vi "Steuerprogramm03-15.vi"() -> ()   [LabVIEW 2010]
uses:
  <vilib>/rvi/interface/nirviReadWriteControl/nirviReadWriteControl.xnode
  <vilib>/rvi/errors/niLvFpgaWhatHappensToTopLevelVI.ctl
  <vilib>/rvi/interface/common/niFpgaNodeNameForErrorReporting.ctl
  <vilib>/rvi/errors/niLvFpgaAdjustHostInterfaceError.vi
  gvbooleschRT.vi
  <vilib>/functionblocks/FB Core/FB Core.xnode
  <vilib>/functionblocks/Counter/Elapsed Timer/Elapsed Timer.vi
  <vilib>/functionblocks/NI_FunctionBlock Libraries.lvlib
  <vilib>/rvi/interface/nirviCloseFPGA/nirviCloseFPGA.xnode
  <vilib>/addons/control/pid/NI_PID_pid.lvlib
  C:/Users/HAGAR-IV/Desktop/Zeugs/Johnny/pertrasgc fpga/FPGA-Programm-10-14.vi
  C:/Users/HAGAR-IV/Desktop/Zeugs/markus/version feb 2012/FPGA Bitfiles/pertrasgcfpga2_FPGATarget_FPGA-Programm-10_16368CB6.lvbitx
  GVMWHorst.vi
  GVMethodenwechsel.vi
  GVHorstSP.vi
  GVZwangs.vi
  GVHK1Hz.vi
  GVHeizenLH.vi
  GVAIs.vi
  <vilib>/addons/control/pid/pid.llb/PID (DBL Array).vi
  GVTrapsMachs.vi
  GVaktuelleTDMS.vi
  GVECDs.vi
  GVZeitenZyklen.vi
  GVProbenvol.vi
  GVVentilposition.vi
  NiFpgaLv.dll
  <vilib>/Utility/error.llb/Error Cluster From Error Code.vi
  <vilib>/Instr/_visa.llb/VISA Configure Serial Port (Instr).vi
  <vilib>/rvi/interface/nirviMethod/nirviMethod.xnode
  GVChroms.vi
  <vilib>/FPGAPlugInAG/cRIO-9114/niLvFpga_Close_cRIO-9114.vi
panel:
  out "AIs3":dbl[](array[numeric])
  out "AIs2":dbl[](array[numeric])
  in  "Tabellarische Darstellung":bool
  out "AIs3":string[](array[string])
  out "AIs2":string[](array[string])
  out "AIs1":string[](array[string])
  out "AIs1":dbl[](array[numeric])
  in  "ServosWarmHigh (us)KaltHigh(us)":T1
  in  "An/Aus":bool
  in  "dargestellte Größe 3":i32(ring)=1 items=["U_WiderstandTrap1 [V]", "TemperaturTrap1 [°C]", "U_WiderstandTrap2 [V]", "TemperaturTrap2 [°C]", "TemperaturMach1 [°C]", "TemperaturMach2 [°C]", "PrC0", "PrC1-Säule2", "PrC1-Säule1", "MFC1-Sample", "MFC1-Methan", "PrC1-BackFlush1", "PrC1-BackFlush2", "MFC2A", "MFC2B", "MFC2C", "PrC2A", "PrC2C", "MFC2D", "MFC2E", "PrC2B"]
  in  "TafelWischen!":bool
  out "schnelleAnzeige":cluster{dbl[], dbl[]}(graph)
  in  "senden":bool
  in  "Schreibpuffer":string
  out "vomLicor":string
  in  "Licor":bool
  in  "SerielleKomm.":bool=TRUE
  in  "ECDSpeichern":bool=TRUE
  in  "HKSpeichern":bool
  in  "Methode speichern":bool
  in  "DetYMax":dbl=100.0
  in  "DetYMin":dbl
  in  "HK2YMax":dbl=100.0
  in  "HK2YMin":dbl
  in  "HK1YMax":dbl=100.0
  in  "HK1YMin":dbl
  out "ZyklusNummernGesamt":i32[](array[numeric])
  in  "Detektor":i32(ring) items=["ECD1", "ECD2"]
  out "Detektor":cluster{dbl[], dbl[]}[](graph)
  out "Zykluslängen [s]":dbl[](array[numeric])
  in  "veränderte Methode benutzen":bool
  in  "Methode verändern":bool
  in  "dargestellte Größe 2":i32(ring)=1 items=["T1-Trap1", "T1-Trap2", "T1-StirlingKühlkopf", "T1-PreCol1", "T1-PreCol2", "T1-MainCol1a", "T1-MainCol1b", "T1-MainCol2a", "T1-MainCol2b", "T1-Bronkhorst1a", "T1-Bronkhorst1b", "T1-Bronkhorst2a", "T1-Bronkhorst2b", "T1-2Pos1B", "T1-Spare9", "T1-2Pos1A", "T1-Spare10", "T1-TurboPump", "T1-StirlingPlatine", "T1-Spare5", "T1-Spare6", "T1-Spare7", "T1-Spare8", "F1-MFM1", "F1-MFM2", "P1-MethaneHP", "P1-MethaneLP", "P1-Vacuum", "TurboSpeed", "I1-MS-AC", "I1-Trap1", "I1-Trap2", "T2-ECD1a", "T2-ECD1b", "T2-ECD2a", "T2-ECD2b", "T2-Col1a", "T2-Col1b", "T2-Col2a", "T2-Col2b", "T2-Spare1", "T2-Spare2", "T2-Oven_a", "T2-Oven_b", "T2-Spare3", "T2-Spare4", "T2-Spare5", "F2-MFM0", "F2-MFM2A", "F2-MFM2B", "P2-N2O_HP", "P2-N2O_LP", "P2-CO2_HP", "P2-CO2_LP", "AI-Spare1", "AI-Spare2", "AI-Spare3", "AI-Spare4", "AI-Spare5", "AI-Spare6", "AI-Spare7", "AI-Spare8", "AI-Spare9", "AI-Spare10", "T0-DC/DC5", "I0-24V_M0", "I0-48V_M1", "I0-24V_M1", "I0-28V_M2", "T0-Drier", "T0-Spare2", "T0-Spare4", "T0-DC/DC7", "I0-20V_Laptop", "I0-28V_M1", "I0-24V_M2", "I0-12V_Licor", "T0-Spare1", "T0-Spare3", "T0-Spare5", "F0-MFM1", "TL-Licor_a", "P0-NitrogenHP", "P0-HeliumHP", "P0-Standard1HP", "P0-Standard2HP", "P0-Standard3HP", "AI-Spare11", "F0-MFM2", "TL-Licor_b", "P0-NitrogenLP", "P0-HeliumLP", "P0-Standard1LP", "P0-Standard2LP", "P0-Standard3LP", "AI-Spare12", "U_WiderstandTrap1 [V]", "TemperaturTrap1 [°C]", "U_WiderstandTrap2 [V]", "TemperaturTrap2 [°C]", "TemperaturMach1 [°C]", "TemperaturMach2 [°C]", "PrC0", "PrC1-Säule2", "PrC1-Säule1", "MFC1-Sample", "MFC1-Methan", "PrC1-BackFlush1", "PrC1-BackFlush2", "MFC2A", "MFC2B", "MFC2C", "PrC2A", "PrC2C", "MFC2D", "MFC2E", "PrC2B"]
  in  "Zeitachse2":i32(ring)=1 items=["Zykluszeit [s] Mod0", "Zykluszeit [s] Mod1", "Zykluszeit [s] Mod2A", "Zykluszeit [s] Mod2B"]
  out "Housekeeping2":cluster{dbl[], dbl[]}(graph)
  out "ZyklusNummern":i32[](array[numeric])
  in  "dargestellte Größe 1":i32(ring)=1 items=["T1-Trap1", "T1-Trap2", "T1-StirlingKühlkopf", "T1-PreCol1", "T1-PreCol2", "T1-MainCol1a", "T1-MainCol1b", "T1-MainCol2a", "T1-MainCol2b", "T1-Bronkhorst1a", "T1-Bronkhorst1b", "T1-Bronkhorst2a", "T1-Bronkhorst2b", "T1-2Pos1B", "T1-Spare9", "T1-2Pos1A", "T1-Spare10", "T1-TurboPump", "T1-StirlingPlatine", "T1-Spare5", "T1-Spare6", "T1-Spare7", "T1-Spare8", "F1-MFM1", "F1-MFM2", "P1-MethaneHP", "P1-MethaneLP", "P1-Vacuum", "TurboSpeed", "I1-MS-AC", "I1-Trap1", "I1-Trap2", "T2-ECD1a", "T2-ECD1b", "T2-ECD2a", "T2-ECD2b", "T2-Col1a", "T2-Col1b", "T2-Col2a", "T2-Col2b", "T2-Spare1", "T2-Spare2", "T2-Oven_a", "T2-Oven_b", "T2-Spare3", "T2-Spare4", "T2-Spare5", "F2-MFM0", "F2-MFM2A", "F2-MFM2B", "P2-N2O_HP", "P2-N2O_LP", "P2-CO2_HP", "P2-CO2_LP", "AI-Spare1", "AI-Spare2", "AI-Spare3", "AI-Spare4", "AI-Spare5", "AI-Spare6", "AI-Spare7", "AI-Spare8", "AI-Spare9", "AI-Spare10", "T0-DC/DC5", "I0-24V_M0", "I0-48V_M1", "I0-24V_M1", "I0-28V_M2", "T0-Drier", "T0-Spare2", "T0-Spare4", "T0-DC/DC7", "I0-20V_Laptop", "I0-28V_M1", "I0-24V_M2", "I0-12V_Licor", "T0-Spare1", "T0-Spare3", "T0-Spare5", "F0-MFM1", "TL-Licor_a", "P0-NitrogenHP", "P0-HeliumHP", "P0-Standard1HP", "P0-Standard2HP", "P0-Standard3HP", "AI-Spare11", "F0-MFM2", "TL-Licor_b", "P0-NitrogenLP", "P0-HeliumLP", "P0-Standard1LP", "P0-Standard2LP", "P0-Standard3LP", "AI-Spare12", "U_WiderstandTrap1 [V]", "TemperaturTrap1 [°C]", "U_WiderstandTrap2 [V]", "TemperaturTrap2 [°C]", "TemperaturMach1 [°C]", "TemperaturMach2 [°C]", "PrC0", "PrC1-Säule2", "PrC1-Säule1", "MFC1-Sample", "MFC1-Methan", "PrC1-BackFlush1", "PrC1-BackFlush2", "MFC2A", "MFC2B", "MFC2C", "PrC2A", "PrC2C", "MFC2D", "MFC2E", "PrC2B"]
  in  "Zeitachse1":i32(ring)=1 items=["Zykluszeit [s] Mod0", "Zykluszeit [s] Mod1", "Zykluszeit [s] Mod2A", "Zykluszeit [s] Mod2B"]
  out "Housekeeping1":cluster{dbl[], dbl[]}(graph)
  out "Big Ben, Methodenzeit, Zykluszeit0, Zykluszeit1, Zykluszeit2A, Zykluszeit2B":i32[](array[numeric])
  in  "global stop RT":bool
  in  "Methode":i32(ring) items=["Leer"]
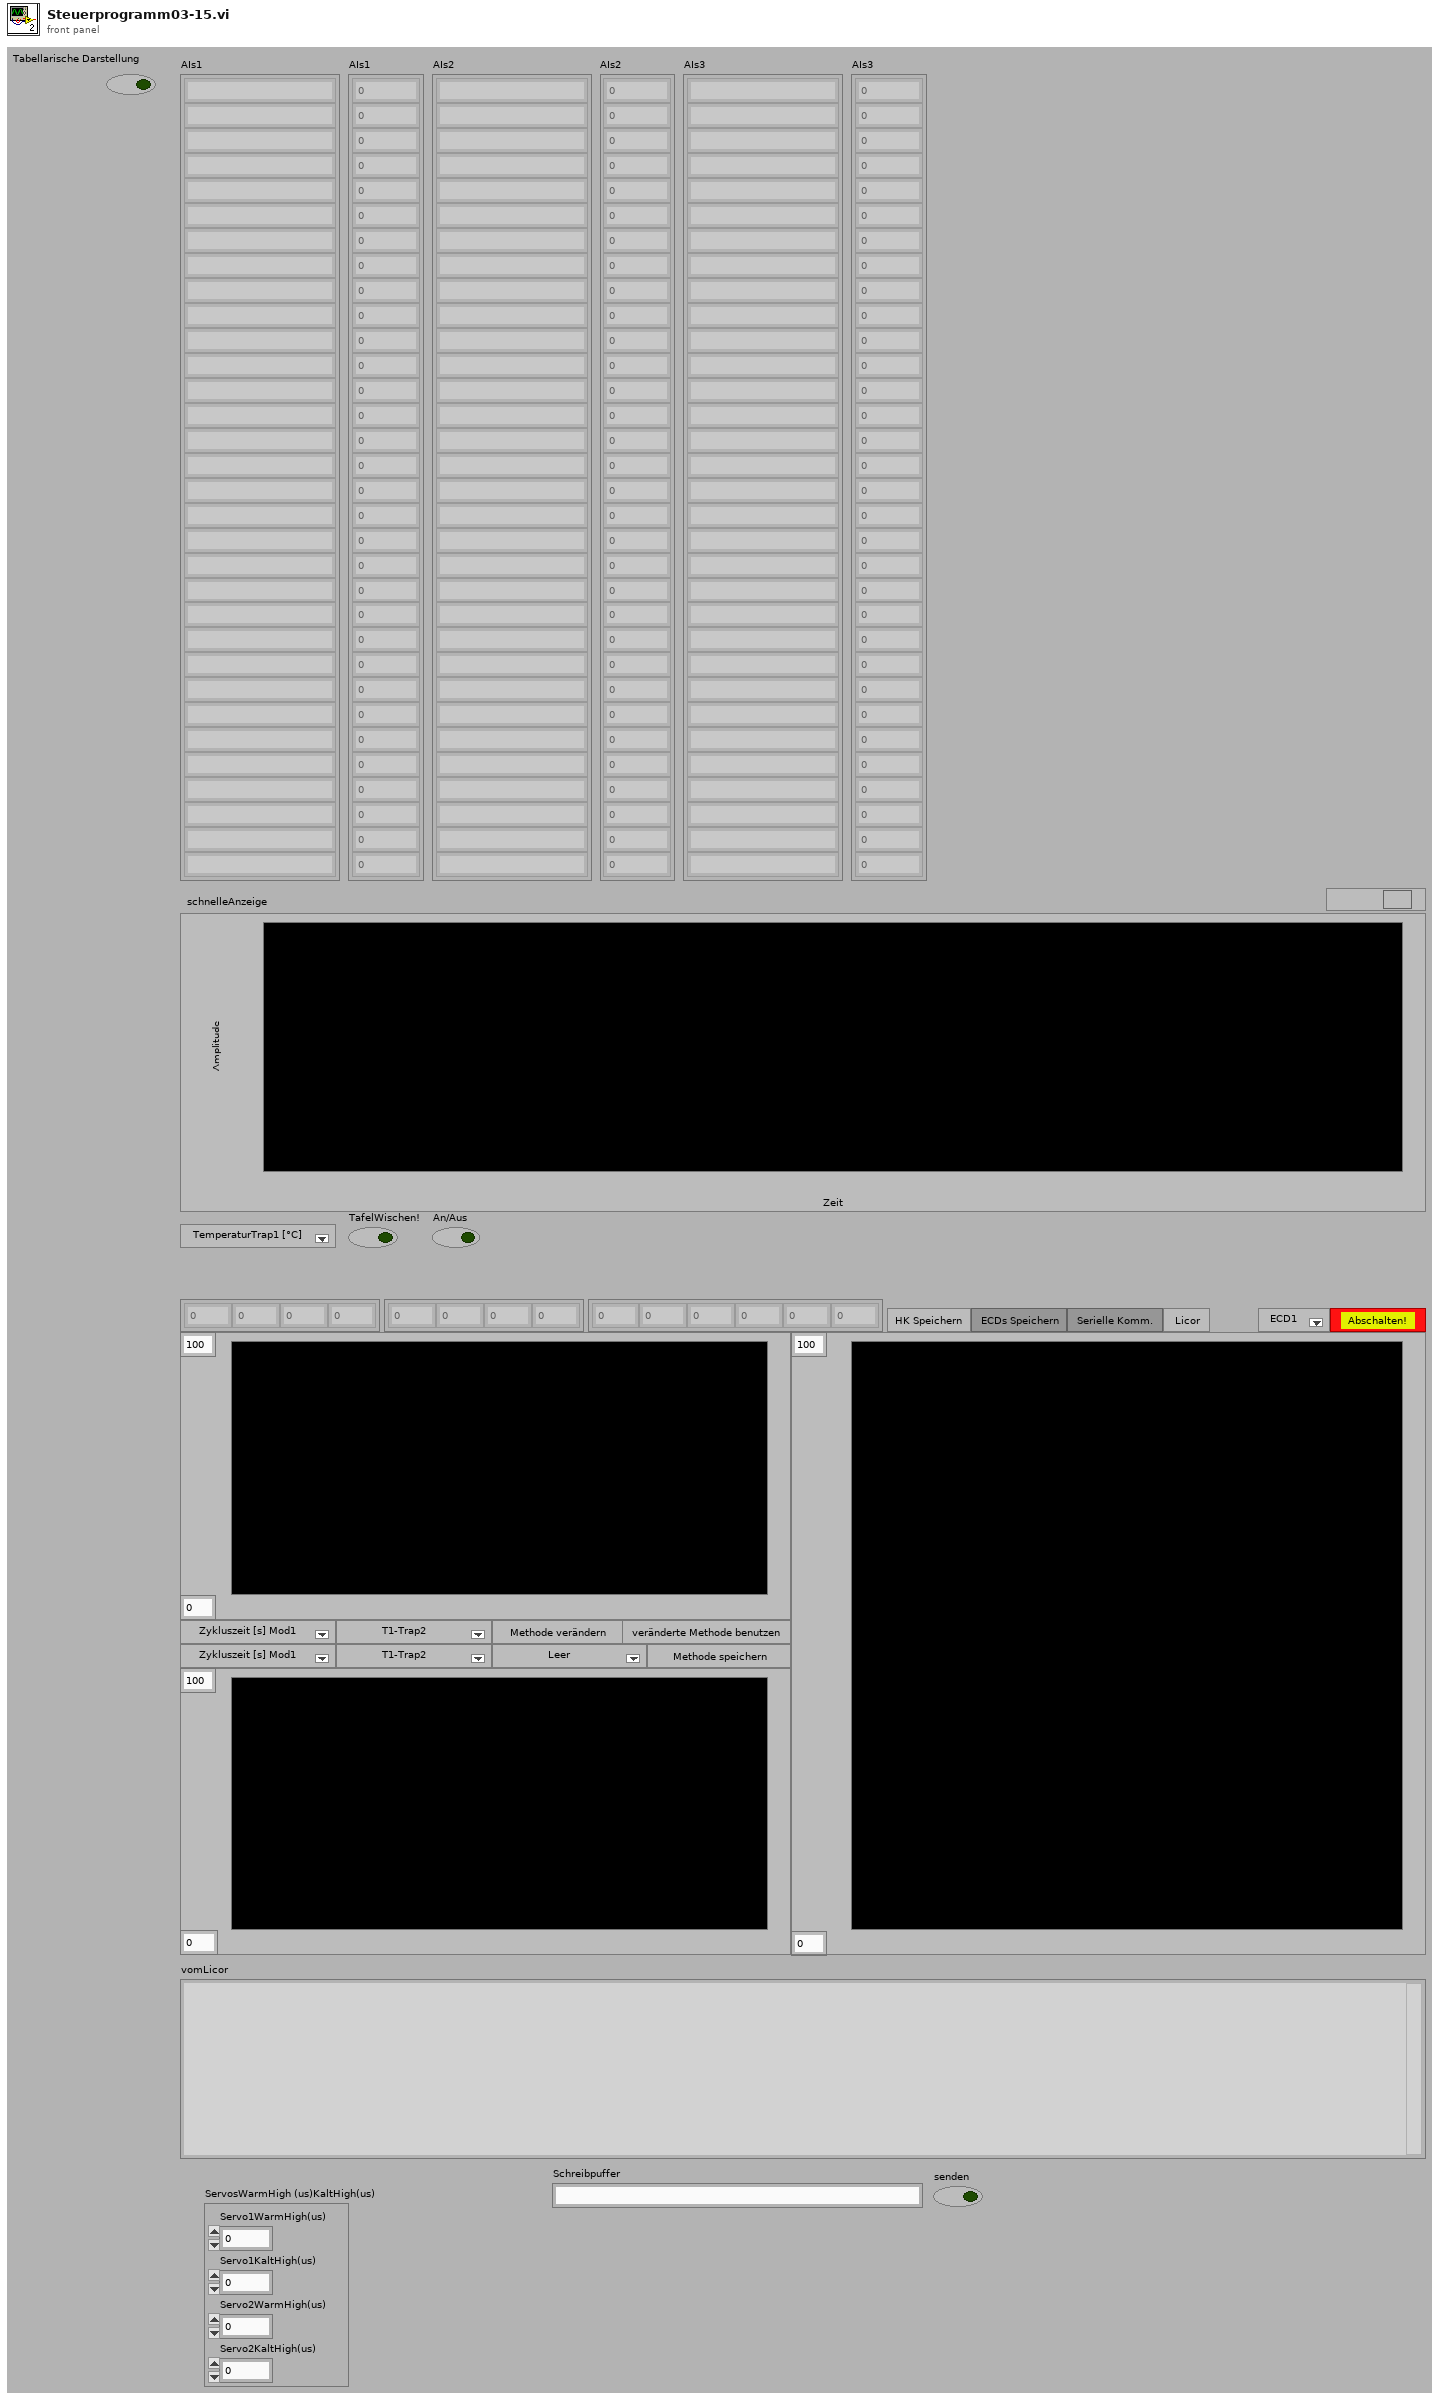
[diagram p1: front panel]
types:
  T1 = cluster{"Servo1WarmHigh(us)":u32, "Servo1KaltHigh(us)":u32, "Servo2WarmHigh(us)":u32, "Servo2KaltHigh(us)":u32}
  T2 = cluster{"Zykluslängen [s]":dbl[], "ZeitpktDIOsMod0":dbl[], "ZeitpktDIOsMod1":dbl[], "ZeitpktDIOsMod2A":dbl[], "ZeitpktDIOsMod2B":dbl[], "DIOsSPMod0":bool[][], "DIOsSPMod1":bool[][], "DIOsSPMod2A":bool[][], "DIOsSPMod2B":bool[][], "Mod0HorstZeitpkt":dbl[], "Mod1HorstZeitpkt":dbl[], "Mod2AHorstZeitpkt":dbl[], "Mod2BHorstZeitpkt":dbl[], "HorstSPMod0":dbl[][], "HorstSPMod1":dbl[][], "HorstSPMod2A":dbl[][], "HorstSPMod2B":dbl[][], "LangsameHeizungenSP":dbl[], "LHHeizen?":bool[], "ZPktFPGABoolesch":dbl[], "FPGABoolesch":bool[][], "ZeitpktFPGAPID":dbl[], "FPGAPID":cluster{"proportional gain (Kc)":fxp<+/-,16,8>, "integral gain (Kc*Ts/Ti)":fxp<+/-,16,8>, "derivative gain (Kc*Td/Ts)":fxp<+/-,16,8>}[][], "ZeitpktFPGAFixp":dbl[], "FPGAFixp":fxp<+/-,16,4>[][], "ZeitpktMach1":dbl[], "TempMach1":dbl[], "ZeitpktMach2":dbl[], "TempMach2":dbl[], "PIDs für \"träge\" Heizungen":cluster{"proportional gain (Kc)":dbl, "integral time (Ti, min)":dbl, "derivative time (Td, min)":dbl}[], "Zwangsbedingungen":dbl[][], "Dateien fürs MS schicken?":bool, "ZeitpunkteMPV":dbl[], "SPMPV":i32[], "ZeitpktMSa":dbl, "ZeitpktMSb":dbl, "Int.Start1":dbl, "Int.Stop1":dbl, "Int.Start2":dbl, "Int.Stop2":dbl, "Methodenname":string}[]
  T3 = cluster{"DIOsMod0Nr":i32[], "DIOsMod1Nr":i32[], "DIOsMod2ANr":i32[], "DIOsMod2BNr":i32[], "AIsLH":i32[], "Anzahl Horst/Modul":i32[], "Regler für den Probenfluß":i32, "StringSPvorgebenMod0":string[], "StringSPvorgebenMod1":string[], "StringSPvorgebenMod2A":string[], "StringSPvorgebenMod2B":string[], "StringMWAntwort0":string[], "StringMWAntwort1":string[], "StringMWAntwort2A":string[], "StringMWAntwort2B":string[], "UmrechnungHorst0":dbl[], "UmrechnungHorst1":dbl[], "UmrechnungHorst2A":dbl[], "UmrechnungHorst2B":dbl[], "StringMWabfragenMod0":string[], "StringMWabfragenMod1":string[], "StringMWabfragenMod2A":string[], "StringMWabfragenMod2B":string[], "Modul1/AI koeff":dbl[][], "Modul2/AI koeff":dbl[][], "Modul3/AI koeff":dbl[][], "Traps/MachsKoeff":dbl[][], "Modul1/AIsNamen":string[], "Modul2/AIsNamen":string[], "Modul3/AIsNamen":string[], "DIOsMod0Name":string[], "DIOsMod1Name":string[], "DIOsMod2AName":string[], "DIOsMod2BName":string[], "HorstMod0Name":string[], "HorstMod1Name":string[], "HorstMod2AName":string[], "HorstMod2BName":string[], "Startmethode":i32, "Dateiordner Housekeeping":path, "Dateiname Housekeeping":string, "DateiordnerECD1":path, "DateinameECD1":string, "DateiordnerECD2":path, "DateinameECD2":string, "NamenLangsameHeizungen":string[], "ModuleLH":i32[]}
  T4 = enum16{"open", "replace", "create", "open or create", "replace or create", "replace or create with confirmation"}
  T5 = cluster{"DIOsMod0Nr":i32[], "DIOsMod1Nr":i32[], "DIOsMod2ANr":i32[], "DIOsMod2BNr":i32[], "AIs für \"träge\" Heizungen":i32[], i32[], "AnschlüsseHorstMod0":enum8{"0", "1", "2", "3", "4", "5", "6", "7", "8"}[], "AnschlüsseHorstMod1":enum8{"0", "1", "2", "3", "4", "5", "6", "7", "8"}[], "AnschlüsseHorstMod2A":enum8{"0", "1", "2", "3", "4", "5", "6", "7", "8"}[], "AnschlüsseHorstMod2B":enum8{"0", "1", "2", "3", "4", "5", "6", "7", "8"}[], "StringSPvorgebenMod0":string[], "StringSPvorgebenMod1":string[], "StringSPvorgebenMod2A":string[], "StringSPvorgebenMod2B":string[], "StringMWAntwort0":string[], "StringMWAntwort1":string[], "StringMWAntwort2A":string[], "StringMWAntwort2B":string[], "UmrechnungHorst0":dbl[], "UmrechnungHorst1":dbl[], "UmrechnungHorst2A":dbl[], "UmrechnungHorst2B":dbl[], "StringMWabfragenMod0":string[], "StringMWabfragenMod1":string[], "StringMWabfragenMod2A":string[], "StringMWabfragenMod2B":string[], "Modul1/AI koeff":dbl[][], "Modul2/AI koeff":dbl[][], "Modul3/AI koeff":dbl[][], "Traps/MachKoeff":dbl[][], "AIsNamen":string[], "DIOsMod0Name":string[], "DIOsMod1Name":string[], "DIOsMod2AName":string[], "DIOsMod2BName":string[], "HorstMod0Name":string[], "HorstMod1Name":string[], "HorstMod2AName":string[], "HorstMod2BName":string[], "Startmethode":i32, "Dateiordner Housekeeping":path, "Dateiname Housekeeping":string, "DateiordnerECD1":path, "DateinameECD1":string, "DateiordnerECD2":path, "DateinameECD2":string}
  T6 = cluster{"Zykluslängen [s]":dbl[], "ZeitpktDIOsMod0":dbl[], "ZeitpktDIOsMod1":dbl[], "ZeitpktDIOsMod2A":dbl[], "ZeitpktDIOsMod2B":dbl[], "DIOsSPMod0":bool[][], "DIOsSPMod1":bool[][], "DIOsSPMod2A":bool[][], "DIOsSPMod2B":bool[][], "Mod0HorstZeitpkt":dbl[], "Mod1HorstZeitpkt":dbl[], "Mod2AHorstZeitpkt":dbl[], "Mod2BHorstZeitpkt":dbl[], "HorstSPMod0":dbl[][], "HorstSPMod1":dbl[][], "HorstSPMod2A":dbl[][], "HorstSPMod2B":dbl[][], "LangsameHeizungenSP":dbl[], "LHHeizen?":bool[], "ZPktFPGABoolesch":dbl[], "FPGABoolesch":bool[][], "ZeitpktFPGAPID":dbl[], "FPGAPID":cluster{"proportional gain (Kc)":fxp<+/-,16,8>, "integral gain (Kc*Ts/Ti)":fxp<+/-,16,8>, "derivative gain (Kc*Td/Ts)":fxp<+/-,16,8>}[][], "ZeitpktFPGAFixp":dbl[], "FPGAFixp":fxp<+/-,16,4>[][], "ZeitpktMach1":dbl[], "TempMach1":dbl[], "ZeitpktMach2":dbl[], "TempMach2":dbl[], "PIDs für \"träge\" Heizungen":cluster{"proportional gain (Kc)":dbl, "integral time (Ti, min)":dbl, "derivative time (Td, min)":dbl}[], "Zwangsbedingungen":dbl[][], "Text0 MS-Datei":string, "Info":string, "wie wird gespeichert?":u16, "Speicherlänge":string, "Dateien fürs MS schicken?":bool, "Pfad MS-Datei CRIO":path}[]
  T7 = cluster{"DIOsMod0Nr":i32[], "DIOsMod1Nr":i32[], "DIOsMod2ANr":i32[], "DIOsMod2BNr":i32[], "AIs für \"träge\" Heizungen":i32[], i32[], "AnschlüsseHorstMod0":enum8{"0", "1", "2", "3", "4", "5", "6", "7", "8"}[], "AnschlüsseHorstMod1":enum8{"0", "1", "2", "3", "4", "5", "6", "7", "8"}[], "AnschlüsseHorstMod2A":enum8{"0", "1", "2", "3", "4", "5", "6", "7", "8"}[], "AnschlüsseHorstMod2B":enum8{"0", "1", "2", "3", "4", "5", "6", "7", "8"}[], "StringSPvorgebenMod0":string[], "StringSPvorgebenMod1":string[], "StringSPvorgebenMod2A":string[], "StringSPvorgebenMod2B":string[], "StringMWAntwort0":string[], "StringMWAntwort1":string[], "StringMWAntwort2A":string[], "StringMWAntwort2B":string[], "UmrechnungHorst0":dbl[], "UmrechnungHorst1":dbl[], "UmrechnungHorst2A":dbl[], "UmrechnungHorst2B":dbl[], "StringMWabfragenMod0":string[], "StringMWabfragenMod1":string[], "StringMWabfragenMod2A":string[], "StringMWabfragenMod2B":string[], "Modul1/AI koeff":dbl[][], "Modul2/AI koeff":dbl[][], "Modul3/AI koeff":dbl[][], "Traps/MachKoeff":dbl[][], "AIsNamen":string[], "DIOsMod0Name":string[], "DIOsMod1Name":string[], "DIOsMod2AName":string[], "DIOsMod2BName":string[], "HorstMod0Name":string[], "HorstMod1Name":string[], "HorstMod2AName":string[], "HorstMod2BName":string[], "Startmethode":i32, "Dateiordner Housekeeping":path, "Dateiname Housekeeping":string}
  T8 = typedef "niFpgaNodeNameForErrorReporting.ctl" = enum16{"Open FPGA VI Reference", "Read/Write Control", "Invoke Method: Abort", "Invoke Method: Acknowledge IRQ", "Invoke Method: Download", "Invoke Method: FIFO.Configure", "Invoke Method: FIFO.Read", "Invoke Method: FIFO.Start", "Invoke Method: FIFO.Stop", "Invoke Method: FIFO.Write", "Invoke Method: Reset", "Invoke Method: Run", "Invoke Method: Wait on IRQ", "Close FPGA VI Reference"}
  T9 = typedef "niLvFpgaWhatHappensToTopLevelVI.ctl" = enum16{"top level VI scripted behind XNode", "top level VI inlined behind XNode"}
  T10 = cluster{"Zyklus1":i32, "Zeitachse1":i32, "dargestellte Größe 1":i32, "Zyklus2":i32, "Zeitachse2":i32, "dargestellte Größe 2":i32}
  T11 = cluster{"DIOsMod0Name":string[], "DIOsMod1Name":string[], "DIOsMod2AName":string[], "DIOsMod2BName":string[], "HorstMod0Name":string[], "HorstMod1Name":string[], "HorstMod2AName":string[], "HorstMod2BName":string[], "NamenLangsameHeizungen":string[]}
  T12 = cluster{"Dateiordner Housekeeping":path, "DateiordnerECD1":path, "DateiordnerECD2":path, "Dateiname Housekeeping":string, "DateinameECD1":string, "DateinameECD2":string, "tdms0":refnum<k34>, "tdms1":refnum<k34>, "tdms0":refnum<k34>, "tdms1":refnum<k34>, "tdms0":refnum<k34>, "tdms1":refnum<k34>}
  T13 = cluster{"Zykluslängen [s]":dbl[], "ZeitpktDIOsMod0":dbl[], "ZeitpktDIOsMod1":dbl[], "ZeitpktDIOsMod2A":dbl[], "ZeitpktDIOsMod2B":dbl[], "DIOsSPMod0":bool[][], "DIOsSPMod1":bool[][], "DIOsSPMod2A":bool[][], "DIOsSPMod2B":bool[][], "Mod0HorstZeitpkt":dbl[], "Mod1HorstZeitpkt":dbl[], "Mod2AHorstZeitpkt":dbl[], "Mod2BHorstZeitpkt":dbl[], "HorstSPMod0":dbl[][], "HorstSPMod1":dbl[][], "HorstSPMod2A":dbl[][], "HorstSPMod2B":dbl[][], "LangsameHeizungenSP":dbl[], "LHHeizen?":bool[], "ZPktFPGABoolesch":dbl[], "FPGABoolesch":bool[][], "ZeitpktFPGAPID":dbl[], "FPGAPID":cluster{"proportional gain (Kc)":fxp<+/-,16,8>, "integral gain (Kc*Ts/Ti)":fxp<+/-,16,8>, "derivative gain (Kc*Td/Ts)":fxp<+/-,16,8>}[][], "ZeitpktFPGAFixp":dbl[], "FPGAFixp":fxp<+/-,16,4>[][], "ZeitpktMach1":dbl[], "TempMach1":dbl[], "ZeitpktMach2":dbl[], "TempMach2":dbl[], "PIDs für \"träge\" Heizungen":cluster{"proportional gain (Kc)":dbl, "integral time (Ti, min)":dbl, "derivative time (Td, min)":dbl}[], "Zwangsbedingungen":dbl[][], "Dateien fürs MS schicken?":bool, "ZeitpunkteMPV":dbl[], "SPMPV":i32[], "ZeitpktMSa":dbl, "ZeitpktMSb":dbl, "Int.Start1":dbl, "Int.Stop1":dbl, "Int.Start2":dbl, "Int.Stop2":dbl, "Methodenname":string}
  T14 = cluster{"proportional gain (Kc)":fxp<+/-,16,8>, "integral gain (Kc*Ts/Ti)":fxp<+/-,16,8>, "derivative gain (Kc*Td/Ts)":fxp<+/-,16,8>}[][]
  T15 = cluster{"proportional gain (Kc)":dbl, "integral time (Ti, min)":dbl, "derivative time (Td, min)":dbl}[]
  T16 = cluster{"Heizen?LH[0]":bool, "Heizen?LH[1]":bool, "Heizen?LH[2]":bool, "Heizen?LH[3]":bool, "Heizen?LH[4]":bool, "Heizen?LH[5]":bool, "Heizen?LH[6]":bool, "Heizen?LH[7]":bool, "Heizen?LH[8]":bool, "Heizen?LH[9]":bool, "Heizen?LH[10]":bool, "Heizen?LH[11]":bool, "Heizen?LH[12]":bool, "Heizen?LH[13]":bool}
  T17 = cluster{"[0]":u32, "[1]":u32, "[2]":u32, "[3]":u32, "[4]":u32, "[5]":u32, "[6]":u32, "[7]":u32, "[8]":u32, "[9]":u32, "[10]":u32, "[11]":u32, "[12]":u32, "[13]":u32}
  T18 = cluster{cluster{"ZeitpktDIOsMod2B":dbl[]}[], cluster{"DIOsSPMod2B":bool[][]}[], cluster{"Mod2BHorstZeitpkt":dbl[]}[], cluster{"HorstSPMod2B":dbl[][]}[], "LHHeizen?":bool[], "ZPktFPGABoolesch":dbl[], "FPGABoolesch":bool[][], "ZeitpktFPGAPID":dbl[], "FPGAPID":cluster{"proportional gain (Kc)":fxp<+/-,16,8>, "integral gain (Kc*Ts/Ti)":fxp<+/-,16,8>, "derivative gain (Kc*Td/Ts)":fxp<+/-,16,8>}[][], "ZeitpktFPGAFixp":dbl[], "FPGAFixp":fxp<+/-,16,4>[][], "ZeitpktMach1":dbl[], "TempMach1":dbl[], "ZeitpktMach2":dbl[], "TempMach2":dbl[], "ZeitpunkteMPV":dbl[], "SPMPV":i32[]}
  T19 = cluster{"ZyklusNummern":i32[], "ZeilennummernDIOs":i32[], "ZwangsDIO?":cluster{bool[]}[], "ZeilennummernHorst":i32[], "ZwangsHorst?":cluster{bool[]}[], "ZeileFPGABoolesch":i32, "ZwangsFPGABoolesch?":bool[], "ZeileFPGAPID":i32, "ZeileFPGAFixp":i32, "ZeileMach1":i32, "ZeileMach2":i32, "ZeilennummerMPV":i32}
  T20 = cluster{"Zyklusnummern 0, 1, 2A, 2B":i32[], i32[], "ZwangsDIO?":cluster{bool[]}[], i32[], "ZwangsHorst?":cluster{bool[]}[], i32, "ZwangsFPGABoolesch?":bool[], i32, i32, i32, i32, "ZeilennummerMPV":i32}
  T21 = cluster{string[], string[], string[], dbl[], dbl[], dbl[]}
  T22 = cluster{"Befehle1":string[], "Befehle2":string[], "Befehle3":string[]}
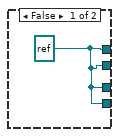
[diagram p2: hidden frame]
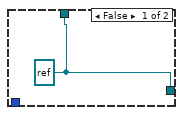
[diagram p3: hidden frame]
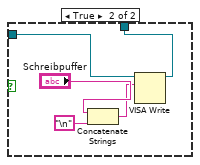
[diagram p6: hidden frame]
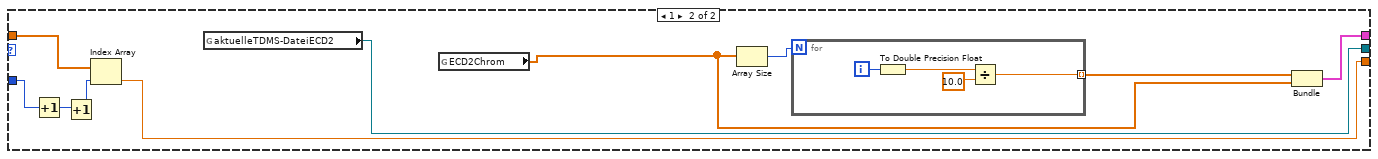
[diagram p15: hidden frame]
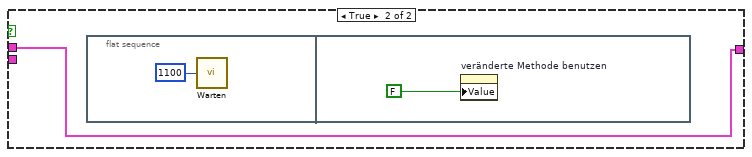
[diagram p16: hidden frame]
diagram:
  (unwired) T5 {"DIOsMod0Nr"=[], "DIOsMod1Nr"=[], "DIOsMod2ANr"=[], "DIOsMod2BNr"=[], "AIs für \"träge\" Heizungen"=[], [], "AnschlüsseHorstMod0"=[], "AnschlüsseHorstMod1"=[], "AnschlüsseHorstMod2A"=[], "AnschlüsseHorstMod2B"=[], "StringSPvorgebenMod0"=[], "StringSPvorgebenMod1"=[], "StringSPvorgebenMod2A"=[], "StringSPvorgebenMod2B"=[], "StringMWAntwort0"=[], "StringMWAntwort1"=[], "StringMWAntwort2A"=[], "StringMWAntwort2B"=[], "UmrechnungHorst0"=[], "UmrechnungHorst1"=[], "UmrechnungHorst2A"=[], "UmrechnungHorst2B"=[], "StringMWabfragenMod0"=[], "StringMWabfragenMod1"=[], "StringMWabfragenMod2A"=[], "StringMWabfragenMod2B"=[], "Modul1/AI koeff"=[], "Modul2/AI koeff"=[], "Modul3/AI koeff"=[], "Traps/MachKoeff"=[], "AIsNamen"=[], "DIOsMod0Name"=[], "DIOsMod1Name"=[], "DIOsMod2AName"=[], "DIOsMod2BName"=[], "HorstMod0Name"=[], "HorstMod1Name"=[], "HorstMod2AName"=[], "HorstMod2BName"=[], "Startmethode"=0, "Dateiordner Housekeeping"=path "", "Dateiname Housekeeping"="", "DateiordnerECD1"=path "", "DateinameECD1"="", "DateiordnerECD2"=path "", "DateinameECD2"=""} ("Einstellungen")
  (unwired) T6 [{"Zykluslängen [s]"=[180.0, 180.0, 180.0, 180.0], "ZeitpktDIOsMod0"=[0.0, 180.0], "ZeitpktDIOsMod1"=[0.0, 2.0, 15.0, 60.0, 61.0, 70.0, 80.0, 170.0, 180.0], "ZeitpktDIOsMod2A"=[0.0, 180.0], "ZeitpktDIOsMod2B"=[0.0, 60.0, 180.0], "DIOsSPMod0"=[[FALSE], [FALSE]], "DIOsSPMod1"=[[TRUE, TRUE, FALSE, TRUE, FALSE, TRUE, TRUE, TRUE, FALSE, FALSE, TRUE, FALSE, FALSE, FALSE, FALSE, FALSE, FALSE, TRUE], [TRUE, FALSE, FALSE, TRUE, FALSE, TRUE, TRUE, TRUE, FALSE, FALSE, TRUE, FALSE, FALSE, FALSE, FALSE, FALSE, FALSE, TRUE], [TRUE, FALSE, FALSE, FALSE, FALSE, TRUE, TRUE, FALSE, FALSE, FALSE, TRUE, FALSE, FALSE, FALSE, FALSE, FALSE, TRUE, TRUE], [TRUE, FALSE, FALSE, FALSE, FALSE, FALSE, TRUE, FALSE, FALSE, FALSE, TRUE, FALSE, FALSE, FALSE, FALSE, FALSE, TRUE, TRUE], [TRUE, FALSE, FALSE, FALSE, FALSE, FALSE, TRUE, FALSE, FALSE, FALSE, TRUE, FALSE, FALSE, FALSE, FALSE, FALSE, TRUE, TRUE], [TRUE, FALSE, FALSE, FALSE, FALSE, FALSE, TRUE, FALSE, FALSE, FALSE, TRUE, FALSE, FALSE, FALSE, FALSE, FALSE, TRUE, TRUE], [TRUE, FALSE, FALSE, FALSE, FALSE, FALSE, TRUE, FALSE, FALSE, FALSE, TRUE, FALSE, FALSE, FALSE, FALSE, FALSE, FALSE, TRUE], [TRUE, FALSE, FALSE, FALSE, FALSE, FALSE, TRUE, FALSE, FALSE, FALSE, TRUE, FALSE, FALSE, FALSE, FALSE, FALSE, FALSE, TRUE], [TRUE, FALSE, FALSE, FALSE, FALSE, FALSE, TRUE, FALSE, FALSE, FALSE, TRUE, FALSE, FALSE, FALSE, FALSE, FALSE, FALSE, TRUE]], "DIOsSPMod2A"=[[FALSE], [FALSE]], "DIOsSPMod2B"=[[FALSE], [FALSE]], "Mod0HorstZeitpkt"=[0.0, 180.0], "Mod1HorstZeitpkt"=[0.0, 55.0, 75.0, 180.0], "Mod2AHorstZeitpkt"=[0.0, 20.0, 180.0], "Mod2BHorstZeitpkt"=[0.0, 380.0], "HorstSPMod0"=[[2.66], [2.66]], "HorstSPMod1"=[[1.9, 0.0, 1.2], [0.0, 0.0, 1.2], [1.9, 0.0, 1.2], [1.9, 0.0, 1.2]], "HorstSPMod2A"=[[300.0], [300.0], [300.0]], "HorstSPMod2B"=[[0.0], [0.0]], "LangsameHeizungenSP"=[60.0, 220.0, 120.0, 60.0, 110.0, 0.0], "LHHeizen?"=[FALSE, TRUE, TRUE, FALSE, TRUE, FALSE], "ZPktFPGABoolesch"=[0.0, 60.0, 75.0, 180.0], "FPGABoolesch"=[[FALSE, FALSE, FALSE, FALSE, TRUE, FALSE], [FALSE, FALSE, TRUE, FALSE, TRUE, FALSE], [FALSE, FALSE, FALSE, FALSE, TRUE, FALSE], [FALSE, FALSE, FALSE, FALSE, TRUE, FALSE]], "ZeitpktFPGAPID"=[0.0, 60.0, 180.0], "FPGAPID"=[[{"proportional gain (Kc)"=5.0, "integral gain (Kc*Ts/Ti)"=0.0, "derivative gain (Kc*Td/Ts)"=0.0}, {"proportional gain (Kc)"=1.0, "integral gain (Kc*Ts/Ti)"=1.66796875, "derivative gain (Kc*Td/Ts)"=0.0}, {"proportional gain (Kc)"=5.0, "integral gain (Kc*Ts/Ti)"=0.03515625, "derivative gain (Kc*Td/Ts)"=0.0234375}, {"proportional gain (Kc)"=1.0, "integral gain (Kc*Ts/Ti)"=1.66796875, "derivative gain (Kc*Td/Ts)"=0.0}], [{"proportional gain (Kc)"=5.0, "integral gain (Kc*Ts/Ti)"=0.0, "derivative gain (Kc*Td/Ts)"=0.0}, {"proportional gain (Kc)"=1.0, "integral gain (Kc*Ts/Ti)"=1.66796875, "derivative gain (Kc*Td/Ts)"=0.0}, {"proportional gain (Kc)"=5.0, "integral gain (Kc*Ts/Ti)"=0.03515625, "derivative gain (Kc*Td/Ts)"=0.0234375}, {"proportional gain (Kc)"=1.0, "integral gain (Kc*Ts/Ti)"=1.66796875, "derivative gain (Kc*Td/Ts)"=0.0}], [{"proportional gain (Kc)"=0.0, "integral gain (Kc*Ts/Ti)"=0.0, "derivative gain (Kc*Td/Ts)"=0.0}, {"proportional gain (Kc)"=0.0, "integral gain (Kc*Ts/Ti)"=0.0, "derivative gain (Kc*Td/Ts)"=0.0}, {"proportional gain (Kc)"=2.0, "integral gain (Kc*Ts/Ti)"=0.03125, "derivative gain (Kc*Td/Ts)"=0.01953125}, {"proportional gain (Kc)"=0.0, "integral gain (Kc*Ts/Ti)"=0.0, "derivative gain (Kc*Td/Ts)"=0.0}], [{"proportional gain (Kc)"=0.0, "integral gain (Kc*Ts/Ti)"=0.0, "derivative gain (Kc*Td/Ts)"=0.0}, {"proportional gain (Kc)"=0.0, "integral gain (Kc*Ts/Ti)"=0.0, "derivative gain (Kc*Td/Ts)"=0.0}, {"proportional gain (Kc)"=2.0, "integral gain (Kc*Ts/Ti)"=0.03125, "derivative gain (Kc*Td/Ts)"=0.01953125}, {"proportional gain (Kc)"=0.0, "integral gain (Kc*Ts/Ti)"=0.0, "derivative gain (Kc*Td/Ts)"=0.0}], [{"proportional gain (Kc)"=0.0, "integral gain (Kc*Ts/Ti)"=0.0, "derivative gain (Kc*Td/Ts)"=0.0}, {"proportional gain (Kc)"=0.0, "integral gain (Kc*Ts/Ti)"=0.0, "derivative gain (Kc*Td/Ts)"=0.0}, {"proportional gain (Kc)"=2.0, "integral gain (Kc*Ts/Ti)"=0.03125, "derivative gain (Kc*Td/Ts)"=0.01953125}, {"proportional gain (Kc)"=0.0, "integral gain (Kc*Ts/Ti)"=0.0, "derivative gain (Kc*Td/Ts)"=0.0}]], "ZeitpktFPGAFixp"=[0.0, 60.0, 75.0, 180.0], "FPGAFixp"=[[0.0, 0.0, 0.0, 0.0, 0.0, 0.0, 2.85009765625, 0.0], [4.59423828125, 4.599365234375, 1.699951171875, 0.0, 0.0, 0.0, 2.85009765625, 0.0], [0.0, 0.0, 0.0, 0.0, 0.0, 0.0, 2.85009765625, 0.0], [0.0, 0.0, 0.0, 0.0, 0.0, 0.0, 2.85009765625, 0.0]], "ZeitpktMach1"=[0.0, 1.0, 100.0, 101.0, 177.0, 178.0, 180.0], "TempMach1"=[50.0, 50.0, 50.0, 250.0, 250.0, 50.0, 50.0], "ZeitpktMach2"=[0.0, 0.0, 120.0], "TempMach2"=[0.0, 0.0, 0.0], "PIDs für \"träge\" Heizungen"=[{"proportional gain (Kc)"=1.0, "integral time (Ti, min)"=0.01, "derivative time (Td, min)"=0.0}, {"proportional gain (Kc)"=2.0, "integral time (Ti, min)"=1.0, "derivative time (Td, min)"=0.0}, {"proportional gain (Kc)"=4.0, "integral time (Ti, min)"=1.0, "derivative time (Td, min)"=0.0}, {"proportional gain (Kc)"=1.0, "integral time (Ti, min)"=0.01, "derivative time (Td, min)"=0.0}, {"proportional gain (Kc)"=2.0, "integral time (Ti, min)"=0.0, "derivative time (Td, min)"=0.0}, {"proportional gain (Kc)"=1.0, "integral time (Ti, min)"=0.01, "derivative time (Td, min)"=0.0}], "Zwangsbedingungen"=[[3.0, 4.0, 100.0, 23.0, 4.0, 200.0, 0.0, 0.0]], "Text0 MS-Datei"="text0", "Info"="info", "wie wird gespeichert?"=0, "Speicherlänge"="100", "Dateien fürs MS schicken?"=FALSE, "Pfad MS-Datei CRIO"=path "c:/"}] ("Eingang 2")
  (unwired) T7 {"DIOsMod0Nr"=[32], "DIOsMod1Nr"=[5, 6, 7, 10, 11, 14, 15, 16, 17, 18, 20, 23, 25, 26, 27, 28, 29, 30], "DIOsMod2ANr"=[33], "DIOsMod2BNr"=[34], "AIs für \"träge\" Heizungen"=[17, 6, 0, 19, 21, 23], [1, 3, 1, 1], "AnschlüsseHorstMod0"=[enum."1"], "AnschlüsseHorstMod1"=[enum."1", enum."1", enum."1"], "AnschlüsseHorstMod2A"=[enum."1"], "AnschlüsseHorstMod2B"=[enum."1"], "StringSPvorgebenMod0"=[":060A020121"], "StringSPvorgebenMod1"=[":060B020121", ":0618020121", ":060D020121"], "StringSPvorgebenMod2A"=[":0519010104"], "StringSPvorgebenMod2B"=[":060C020121 "], "StringMWAntwort0"=[":060A020121"], "StringMWAntwort1"=[":060B020121", ":0618020121", ":060D020121"], "StringMWAntwort2A"=[":0619020121"], "StringMWAntwort2B"=[":060C020121"], "UmrechnungHorst0"=[0.0003125], "UmrechnungHorst1"=[9.375e-05, 9.375e-05, 9.375e-05], "UmrechnungHorst2A"=[1.0], "UmrechnungHorst2B"=[9.375e-05], "StringMWabfragenMod0"=[":060A0401210120"], "StringMWabfragenMod1"=[":060B0401210120", ":06180401210120", ":060D0401210120"], "StringMWabfragenMod2A"=[":06190401210120"], "StringMWabfragenMod2B"=[":060C0401210120"], "Modul1/AI koeff"=[[-249.333, 111.873, 2.1471], [-249.333, 111.873, 2.1471], [-249.333, 111.873, 2.1471], [-249.333, 111.873, 2.1471], [-237.2852, -153.162, 6.0782], [-237.2852, -153.162, 6.0782], [-249.333, 111.873, 2.1471], [-249.333, 111.873, 2.1471], [-249.333, 111.873, 2.1471], [-249.333, 111.873, 2.1471], [-249.333, 111.873, 2.1471], [-249.333, 111.873, 2.1471], [-249.333, 111.873, 2.1471], [-249.333, 111.873, 2.1471], [-249.333, 111.873, 2.1471], [0.0, 1.0, 0.0], [-249.333, 111.873, 2.1471], [-249.333, 111.873, 2.1471], [-249.333, 111.873, 2.1471], [-249.333, 111.873, 2.1471], [-249.333, 111.873, 2.1471], [-249.333, 111.873, 2.1471], [-249.333, 111.873, 2.1471], [-249.333, 111.873, 2.1471], [0.0, 1.0, 0.0], [0.0, 1.0, 0.0], [0.0, 1.0, 0.0], [0.0, 1.0, 0.0], [0.0, 1.0, 0.0], [0.0, 1.0, 0.0], [0.0, 1.0, 0.0], [0.0, 1.0, 0.0]], "Modul2/AI koeff"=[[0.0, 1.0, 0.0], [0.0, 1.0, 0.0], [0.0, 1.0, 0.0], [0.0, 1.0, 0.0], [0.0, 1.0, 0.0], [0.0, 1.0, 0.0], [0.0, 1.0, 0.0], [0.0, 1.0, 0.0], [0.0, 1.0, 0.0], [0.0, 1.0, 0.0], [0.0, 1.0, 0.0], [0.0, 1.0, 0.0], [0.0, 1.0, 0.0], [0.0, 1.0, 0.0], [0.0, 1.0, 0.0], [0.0, 1.0, 0.0], [0.0, 1.0, 0.0], [0.0, 1.0, 0.0], [0.0, 1.0, 0.0], [0.0, 1.0, 0.0], [0.0, 1.0, 0.0], [0.0, 1.0, 0.0], [0.0, 1.0, 0.0], [0.0, 1.0, 0.0], [0.0, 1.0, 0.0], [0.0, 1.0, 0.0], [0.0, 1.0, 0.0], [0.0, 1.0, 0.0], [0.0, 1.0, 0.0], [0.0, 1.0, 0.0], [0.0, 1.0, 0.0], [0.0, 1.0, 0.0]], "Modul3/AI koeff"=[[0.0, 1.0, 0.0], [0.0, 1.0, 0.0], [0.0, 1.0, 0.0], [0.0, 1.0, 0.0], [0.0, 1.0, 0.0], [0.0, 1.0, 0.0], [0.0, 1.0, 0.0], [0.0, 1.0, 0.0], [0.0, 1.0, 0.0], [0.0, 1.0, 0.0], [0.0, 1.0, 0.0], [0.0, 1.0, 0.0], [0.0, 1.0, 0.0], [0.0, 1.0, 0.0], [0.0, 1.0, 0.0], [0.0, 1.0, 0.0], [0.0, 1.0, 0.0], [0.0, 1.0, 0.0], [0.0, 1.0, 0.0], [0.0, 1.0, 0.0], [0.0, 1.0, 0.0], [0.0, 1.0, 0.0], [0.0, 1.0, 0.0], [0.0, 1.0, 0.0], [0.0, 1.0, 0.0], [0.0, 1.0, 0.0], [0.0, 1.0, 0.0], [0.0, 1.0, 0.0], [0.0, 1.0, 0.0], [0.0, 1.0, 0.0], [0.0, 1.0, 0.0], [0.0, 1.0, 0.0]], "Traps/MachKoeff"=[[0.0, 1.0, 0.0], [-249.333, 111.873, 2.1471], [0.0, 1.0, 0.0], [-249.333, 111.873, 2.1471], [-237.2852, 153.1621, 6.0782], [-237.2852, 153.1621, 6.0782]], "AIsNamen"=["T-MainCol3", "T-Trap1", "T-Trap2", "T-Stirling", "T-PreCol1", "T-PreCol2", "T-MainCol1", "T-MainCol2", "T-T-Line2", "T-MI1", "T-MI2", "T-MI3", "T-MI4", "T-MI5", "T-MI6", "F-MFM1", "T-MainCol4", "T-BHorst1", "T-BHorst2", "T-BHorst3", "T-BHorst4", "T-Oven1", "T-Oven2", "T-T-Line1", "F-MFM2", "P-Me-HP", "P-Me-LP", "P-Vac", "Ref-Turbo", "I-MS-AC", "I-Trap1", "I-Trap2", "Mod2/AI0", "Mod2/AI1", "Mod2/AI2", "Mod2/AI3", "Mod2/AI4", "Mod2/AI5", "Mod2/AI6", "Mod2/AI7", "Mod2/AI8", "Mod2/AI9", "Mod2/AI10", "Mod2/AI11", "Mod2/AI12", "Mod2/AI13", "Mod2/AI14", "Mod2/AI15", "Mod2/AI16", "Mod2/AI17", "Mod2/AI18", "Mod2/AI19", "Mod2/AI20", "Mod2/AI21", "Mod2/AI22", "Mod2/AI23", "Mod2/AI24", "Mod2/AI25", "Mod2/AI26", "Mod2/AI27", "Mod2/AI28", "Mod2/AI29", "Mod2/AI30", "Mod2/AI31", "Mod3/AI0", "Mod3/AI1", "Mod3/AI2", "Mod3/AI3", "Mod3/AI4", "Mod3/AI5", "Mod3/AI6", "Mod3/AI7", "Mod3/AI8", "Mod3/AI9", "Mod3/AI10", "Mod3/AI11", "Mod3/AI12", "Mod3/AI13", "Mod3/AI14", "Mod3/AI15", "Mod3/AI16", "Mod3/AI17", "Mod3/AI18", "Mod3/AI19", "Mod3/AI20", "Mod3/AI21", "Mod3/AI22", "Mod3/AI23", "Mod3/AI24", "Mod3/AI25", "Mod3/AI26", "Mod3/AI27", "Mod3/AI28", "Mod3/AI29", "Mod3/AI30", "Mod3/AI31"], "DIOsMod0Name"=["blindDIO0"], "DIOsMod1Name"=["on/off P-MS", "MS Start", "MS Stop", "FanMach1", "FanReserve", "Valve1A", "on/off PrePump", "Air-In", "on/off VacP2", "on/off VacP1", "S1D", "FanMach2", "S1C", "on/off Stirling", "S1B", "S1A", "Valve1B", "on/off Turbo"], "DIOsMod2AName"=["blindDIO2A"], "DIOsMod2BName"=["blindDIO2B"], "HorstMod0Name"=["MFC1B"], "HorstMod1Name"=["PressContr1A", "PressContr1B", "PressContr1C"], "HorstMod2AName"=["MFC1A"], "HorstMod2BName"=["PressContr1D"], "Startmethode"=0, "Dateiordner Housekeeping"=path "C:/data", "Dateiname Housekeeping"="test"} ("Einstellungen")
  (unwired) T7 {"DIOsMod0Nr"=[32], "DIOsMod1Nr"=[5, 6, 7, 10, 11, 14, 15, 16, 17, 18, 20, 23, 25, 26, 27, 28, 29, 30], "DIOsMod2ANr"=[33], "DIOsMod2BNr"=[34], "AIs für \"träge\" Heizungen"=[17, 6, 0, 19, 21, 23], [1, 3, 1, 1], "AnschlüsseHorstMod0"=[enum."1"], "AnschlüsseHorstMod1"=[enum."1", enum."1", enum."1"], "AnschlüsseHorstMod2A"=[enum."1"], "AnschlüsseHorstMod2B"=[enum."1"], "StringSPvorgebenMod0"=[":060A020121"], "StringSPvorgebenMod1"=[":060B020121", ":0618020121", ":060D020121"], "StringSPvorgebenMod2A"=[":0619020121"], "StringSPvorgebenMod2B"=[":060C020121"], "StringMWAntwort0"=[":060A020121"], "StringMWAntwort1"=[":060B020121", ":0618020121", ":060D020121"], "StringMWAntwort2A"=[":0619020121"], "StringMWAntwort2B"=[":060C020121"], "UmrechnungHorst0"=[0.0003125], "UmrechnungHorst1"=[9.375e-05, 9.375e-05, 9.375e-05], "UmrechnungHorst2A"=[0.046875], "UmrechnungHorst2B"=[9.375e-05], "StringMWabfragenMod0"=[":060A0401210120"], "StringMWabfragenMod1"=[":060B0401210120", ":06180401210120", ":060D0401210120"], "StringMWabfragenMod2A"=[":06190401210120"], "StringMWabfragenMod2B"=[":060C0401210120"], "Modul1/AI koeff"=[[-249.333, 111.873, 2.1471], [-249.333, 111.873, 2.1471], [-249.333, 111.873, 2.1471], [-249.333, 111.873, 2.1471], [-237.2852, -153.162, 6.0782], [-237.2852, -153.162, 6.0782], [-249.333, 111.873, 2.1471], [-249.333, 111.873, 2.1471], [-249.333, 111.873, 2.1471], [-249.333, 111.873, 2.1471], [-249.333, 111.873, 2.1471], [-249.333, 111.873, 2.1471], [-249.333, 111.873, 2.1471], [-249.333, 111.873, 2.1471], [-249.333, 111.873, 2.1471], [0.0, 1.0, 0.0], [-249.333, 111.873, 2.1471], [-249.333, 111.873, 2.1471], [-249.333, 111.873, 2.1471], [-249.333, 111.873, 2.1471], [-249.333, 111.873, 2.1471], [-249.333, 111.873, 2.1471], [-249.333, 111.873, 2.1471], [-249.333, 111.873, 2.1471], [0.0, 1.0, 0.0], [0.0, 1.0, 0.0], [0.0, 1.0, 0.0], [0.0, 1.0, 0.0], [0.0, 1.0, 0.0], [0.0, 1.0, 0.0], [0.0, 1.0, 0.0], [0.0, 1.0, 0.0]], "Modul2/AI koeff"=[[0.0, 1.0, 0.0], [0.0, 1.0, 0.0], [0.0, 1.0, 0.0], [0.0, 1.0, 0.0], [0.0, 1.0, 0.0], [0.0, 1.0, 0.0], [0.0, 1.0, 0.0], [0.0, 1.0, 0.0], [0.0, 1.0, 0.0], [0.0, 1.0, 0.0], [0.0, 1.0, 0.0], [0.0, 1.0, 0.0], [0.0, 1.0, 0.0], [0.0, 1.0, 0.0], [0.0, 1.0, 0.0], [0.0, 1.0, 0.0], [0.0, 1.0, 0.0], [0.0, 1.0, 0.0], [0.0, 1.0, 0.0], [0.0, 1.0, 0.0], [0.0, 1.0, 0.0], [0.0, 1.0, 0.0], [0.0, 1.0, 0.0], [0.0, 1.0, 0.0], [0.0, 1.0, 0.0], [0.0, 1.0, 0.0], [0.0, 1.0, 0.0], [0.0, 1.0, 0.0], [0.0, 1.0, 0.0], [0.0, 1.0, 0.0], [0.0, 1.0, 0.0], [0.0, 1.0, 0.0]], "Modul3/AI koeff"=[[0.0, 1.0, 0.0], [0.0, 1.0, 0.0], [0.0, 1.0, 0.0], [0.0, 1.0, 0.0], [0.0, 1.0, 0.0], [0.0, 1.0, 0.0], [0.0, 1.0, 0.0], [0.0, 1.0, 0.0], [0.0, 1.0, 0.0], [0.0, 1.0, 0.0], [0.0, 1.0, 0.0], [0.0, 1.0, 0.0], [0.0, 1.0, 0.0], [0.0, 1.0, 0.0], [0.0, 1.0, 0.0], [0.0, 1.0, 0.0], [0.0, 1.0, 0.0], [0.0, 1.0, 0.0], [0.0, 1.0, 0.0], [0.0, 1.0, 0.0], [0.0, 1.0, 0.0], [0.0, 1.0, 0.0], [0.0, 1.0, 0.0], [0.0, 1.0, 0.0], [0.0, 1.0, 0.0], [0.0, 1.0, 0.0], [0.0, 1.0, 0.0], [0.0, 1.0, 0.0], [0.0, 1.0, 0.0], [0.0, 1.0, 0.0], [0.0, 1.0, 0.0], [0.0, 1.0, 0.0]], "Traps/MachKoeff"=[[0.0, 1.0, 0.0], [-249.333, 111.873, 2.1471], [0.0, 1.0, 0.0], [-249.333, 111.873, 2.1471], [-237.2852, 153.1621, 6.0782], [-237.2852, 153.1621, 6.0782]], "AIsNamen"=["T-MainCol3", "T-Trap1", "T-Trap2", "T-Stirling", "T-PreCol1", "T-PreCol2", "T-MainCol1", "T-MainCol2", "T-T-Line2", "T-MI1", "T-MI2", "T-MI3", "T-MI4", "T-MI5", "T-MI6", "F-MFM1", "T-MainCol4", "T-BHorst1", "T-BHorst2", "T-BHorst3", "T-BHorst4", "T-Oven1", "T-Oven2", "T-T-Line1", "F-MFM2", "P-Me-HP", "P-Me-LP", "P-Vac", "Ref-Turbo", "I-MS-AC", "I-Trap1", "I-Trap2", "Mod2/AI0", "Mod2/AI1", "Mod2/AI2", "Mod2/AI3", "Mod2/AI4", "Mod2/AI5", "Mod2/AI6", "Mod2/AI7", "Mod2/AI8", "Mod2/AI9", "Mod2/AI10", "Mod2/AI11", "Mod2/AI12", "Mod2/AI13", "Mod2/AI14", "Mod2/AI15", "Mod2/AI16", "Mod2/AI17", "Mod2/AI18", "Mod2/AI19", "Mod2/AI20", "Mod2/AI21", "Mod2/AI22", "Mod2/AI23", "Mod2/AI24", "Mod2/AI25", "Mod2/AI26", "Mod2/AI27", "Mod2/AI28", "Mod2/AI29", "Mod2/AI30", "Mod2/AI31", "Mod3/AI0", "Mod3/AI1", "Mod3/AI2", "Mod3/AI3", "Mod3/AI4", "Mod3/AI5", "Mod3/AI6", "Mod3/AI7", "Mod3/AI8", "Mod3/AI9", "Mod3/AI10", "Mod3/AI11", "Mod3/AI12", "Mod3/AI13", "Mod3/AI14", "Mod3/AI15", "Mod3/AI16", "Mod3/AI17", "Mod3/AI18", "Mod3/AI19", "Mod3/AI20", "Mod3/AI21", "Mod3/AI22", "Mod3/AI23", "Mod3/AI24", "Mod3/AI25", "Mod3/AI26", "Mod3/AI27", "Mod3/AI28", "Mod3/AI29", "Mod3/AI30", "Mod3/AI31"], "DIOsMod0Name"=["blindDIO0"], "DIOsMod1Name"=["on/off P-MS", "MS Start", "MS Stop", "FanMach1", "FanReserve", "Valve1A", "on/off PrePump", "S1Reserve", "on/off VacP2", "on/off VacP1", "S1D", "FanMach2", "S1C", "on/off Stirling", "S1B", "S1A", "Valve1B", "on/off Turbo"], "DIOsMod2AName"=["blindDIO2A"], "DIOsMod2BName"=["blindDIO2B"], "HorstMod0Name"=["MFC1B"], "HorstMod1Name"=["PressContr1A", "PressContr1B", "PressContr1C"], "HorstMod2AName"=["MFC1A"], "HorstMod2BName"=["PressContr1D"], "Startmethode"=0, "Dateiordner Housekeeping"=path "C:/", "Dateiname Housekeeping"="test"} ("Einstellungen")
  n1 = Open/Create/Replace File(file path (use dialog)=path "c:/einstellungen.per" ("Datei (Dialog verwenden)"), operation (0:open)=T4."open" ("Operation (0:Öffnen)")) -> (refnum out=w11:refnum<file>)  [unwired: 4 in, 2 out]
  n2 = Read from Binary File(5:T3 {"DIOsMod0Nr"=[], "DIOsMod1Nr"=[], "DIOsMod2ANr"=[], "DIOsMod2BNr"=[], "AIsLH"=[], "Anzahl Horst/Modul"=[], "Regler für den Probenfluß"=0, "StringSPvorgebenMod0"=[], "StringSPvorgebenMod1"=[], "StringSPvorgebenMod2A"=[], "StringSPvorgebenMod2B"=[], "StringMWAntwort0"=[], "StringMWAntwort1"=[], "StringMWAntwort2A"=[], "StringMWAntwort2B"=[], "UmrechnungHorst0"=[], "UmrechnungHorst1"=[], "UmrechnungHorst2A"=[], "UmrechnungHorst2B"=[], "StringMWabfragenMod0"=[], "StringMWabfragenMod1"=[], "StringMWabfragenMod2A"=[], "StringMWabfragenMod2B"=[], "Modul1/AI koeff"=[], "Modul2/AI koeff"=[], "Modul3/AI koeff"=[], "Traps/MachsKoeff"=[], "Modul1/AIsNamen"=[], "Modul2/AIsNamen"=[], "Modul3/AIsNamen"=[], "DIOsMod0Name"=[], "DIOsMod1Name"=[], "DIOsMod2AName"=[], "DIOsMod2BName"=[], "HorstMod0Name"=[], "HorstMod1Name"=[], "HorstMod2AName"=[], "HorstMod2BName"=[], "Startmethode"=0, "Dateiordner Housekeeping"=path "", "Dateiname Housekeeping"="", "DateiordnerECD1"=path "", "DateinameECD1"="", "DateiordnerECD2"=path "", "DateinameECD2"="", "NamenLangsameHeizungen"=[], "ModuleLH"=[]} ("Einstellungen"), 11:w11) -> (2:w9:T3, 3:w10:refnum<file>)  [unwired: 4 in, 2 out]
  n3 = Close File(refnum=w10) -> ()  [unwired: 1 in, 2 out]
  n4 = flat-sequence {
    tunnel: [w169] -> w39
    tunnel: [w97] -> w38
    tunnel: [w193] -> w36
    tunnel: [w190] -> w35
    tunnel: [w192] -> w34
    tunnel: [w184] -> w33
    tunnel: [w191] -> w32
    tunnel: [w101] -> w31
    tunnel: [w183] -> w30
    tunnel: [w182] -> w29
    tunnel: [w176] -> w28
    tunnel: [w104] -> w27
    tunnel: [w74] -> w26
    tunnel: [w189] -> w25
    tunnel: [w181] -> w24
    tunnel: [w180] -> w23
    tunnel: [w172] -> w22
    tunnel: [w171] -> w21
    tunnel: [w170] -> w20
    tunnel: [w168] -> w19
    tunnel: [w167] -> w18
    tunnel: [w166] -> w17
    tunnel: [w163] -> w16
    tunnel: [w145] -> w15
    tunnel: w9 -> [w100]
    tunnel: [w143] -> w14
    tunnel: w3 -> [w144]
    tunnel: [w97] -> w1
    tunnel: w39 -> [w254]
    tunnel: w38 -> [w330]
    tunnel: [w254] -> w37
    tunnel: w36 -> [_]
    tunnel: w35 -> [w285]
    tunnel: w34 -> [w284]
    tunnel: w33 -> [w286]
    tunnel: w32 -> [w283]
    tunnel: w31 -> [w258]
    tunnel: w30 -> [w253]
    tunnel: w29 -> [w248]
    tunnel: w28 -> [w245]
    tunnel: w27 -> [w246]
    tunnel: w26 -> [w249]
    tunnel: w25 -> [w328]
    tunnel: w24 -> [w256]
    tunnel: w23 -> [w329]
    tunnel: w22 -> [w326]
    tunnel: w21 -> [w325]
    tunnel: w20 -> [w324]
    tunnel: w19 -> [w323]
    tunnel: w18 -> [w322]
    tunnel: w17 -> [w321]
    tunnel: w16 -> [w275]
    tunnel: w15 -> [w257]
    tunnel: w14 -> [w244]
    tunnel: w3 -> [w243]
    tunnel: w1 -> [w241]
    tunnel: w37 -> [w1195]
    frame #0 {
      w56 = 0.0 ("Probenvol.1")
      w63 = dbl[] [-1.0] ("ECD1MW")
      w64 = FALSE ("ECD1Empfangen?")
      w54 = string[] ["U_WiderstandTrap1 [V]", "TemperaturTrap1 [°C]", "U_WiderstandTrap2 [V]", "TemperaturTrap2 [°C]", "TemperaturMach1 [°C]", "TemperaturMach2 [°C]"]
      w187 = string[] ["Big Ben [s]", "Methodenzeit [s]", "Zykluszeit [s] Mod0", "Zykluszeit [s] Mod1", "Zykluszeit [s] Mod2A", "Zykluszeit [s] Mod2B"]
      w177 = FALSE ("Undefinierte Werte möglich")
      w178 = FALSE ("global stop RT")
      n5 = Unbundle(w100) -> ("DIOsMod0Nr"=w84:i32[], "DIOsMod1Nr"=w83:i32[], "DIOsMod2ANr"=w82:i32[], "DIOsMod2BNr"=w81:i32[], "AIsLH"=w71:i32[], "Anzahl Horst/Modul"=w74:i32[], "Regler für den Probenfluß"=w143:i32, "StringSPvorgebenMod0"=w142:string[], "StringSPvorgebenMod1"=w141:string[], "StringSPvorgebenMod2A"=w140:string[], "StringSPvorgebenMod2B"=w139:string[], "StringMWAntwort0"=w138:string[], "StringMWAntwort1"=w137:string[], "StringMWAntwort2A"=w136:string[], "StringMWAntwort2B"=w135:string[], "UmrechnungHorst0"=w134:dbl[], "UmrechnungHorst1"=w133:dbl[], "UmrechnungHorst2A"=w132:dbl[], "UmrechnungHorst2B"=w131:dbl[], "StringMWabfragenMod0"=w130:string[], "StringMWabfragenMod1"=w129:string[], "StringMWabfragenMod2A"=w128:string[], "StringMWabfragenMod2B"=w127:string[], "Modul1/AI koeff"=w126:dbl[][], "Modul2/AI koeff"=w125:dbl[][], "Modul3/AI koeff"=w124:dbl[][], "Traps/MachsKoeff"=w123:dbl[][], "Modul1/AIsNamen"=w122:string[], "Modul2/AIsNamen"=w121:string[], "Modul3/AIsNamen"=w120:string[], "DIOsMod0Name"=w119:string[], "DIOsMod1Name"=w118:string[], "DIOsMod2AName"=w117:string[], "DIOsMod2BName"=w116:string[], "HorstMod0Name"=w115:string[], "HorstMod1Name"=w114:string[], "HorstMod2AName"=w113:string[], "HorstMod2BName"=w112:string[], "Startmethode"=w97:i32, "Dateiordner Housekeeping"=w111:path, "Dateiname Housekeeping"=w110:string, "DateiordnerECD1"=w109:path, "DateinameECD1"=w108:string, "DateiordnerECD2"=w107:path, "DateinameECD2"=w106:string, "NamenLangsameHeizungen"=w105:string[], "ModuleLH"=w99:i32[])
      n6 = global write "gvbooleschRT.vi" "global stop RT"(w178) -> ()
      n7 = Decrement(x=w99) -> (x-1=w98:i32[])
      n8 = Multiply(x=w98, y=32) -> (x*y=w102:i32[])
      n9 = property on="dargestellte Größe 2" class="Ring (strict)"("AllowUndefVals"=w177) -> ()  [unwired: 2 in, 2 out]
      n10 = property on="Zeitachse2" class="Ring (strict)"("AllowUndefVals"=w177) -> ()  [unwired: 2 in, 2 out]
      n11 = property on="Zeitachse1" class="Ring (strict)"("AllowUndefVals"=w177) -> ()  [unwired: 2 in, 2 out]
      n12 = property on="dargestellte Größe 1" class="Ring (strict)"("AllowUndefVals"=w177) -> ()  [unwired: 2 in, 2 out]
      n13 = property on="Methode" class="Ring (strict)"("AllowUndefVals"=w177) -> ()  [unwired: 2 in, 2 out]
      n14 = property on="Methode" class="Ring (strict)"("Value"=w97) -> ()  [unwired: 2 in, 2 out]
      n15 = Add(x=w102, y=w71) -> (x+y=w101:i32[])
      n16 = Add Array Elements(numeric array=w74) -> (sum=w86:i32)
      n17 = for {
        tunnel: [w221] -> w185 mode=indexing
        tunnel: w144 -> [w222] mode=indexing
        n18 = Unbundle(w222) -> ("Methodenname"=w221:string)  [unwired: 40 out]
      }
      n19 = global write "GVProbenvol.vi" "Probenvol.2"(w56) -> ()
      n20 = global write "GVProbenvol.vi" "Probenvol.1"(w56) -> ()
      n21 = local write "global stop RT"(w178) -> ()
      n22 = Initialize Array(0.0 ("Element"), w86) -> (w85:dbl[])
      n23 = Initialize Array(-1.0, w86) -> (w88:dbl[])
      n24 = Initialize Array(-1.0 ("Element"), 96 ("Dimension")) -> (w68:dbl[])
      n25 = Initialize Array(-1.0 ("Element"), 6 ("Dimension")) -> (w67:dbl[])
      n26 = call "FPGA-Start.vi"("ServosWarmHigh (us)KaltHigh(us)"="ServosWarmHigh (us)KaltHigh(us)") -> ("error out"=w193:errorcluster, "FPGA VI Reference Out"=w169:refnum<k20>)  [unwired: 1 in]
      n27 = global write "GVMWHorst.vi" "MWHorst"(w88) -> ()
      n28 = global write "GVHorstSP.vi" "HorstSP"(w85) -> ()
      n29 = global write "GVMethodenwechsel.vi" "Methodenwechsel?"(FALSE ("Methodenwechsel?")) -> ()
      n30 = global write "GVTrapsMachs.vi" "Traps/Machs"(w67) -> ()
      n31 = Build Array (concatenate)(w68, w67) -> (w66:dbl[])
      n32 = Build Array(w84, w83, w82, w81) -> (w80:i32[][])
      n33 = Build Array (concatenate)(w122, w121, w120) -> (w43:string[])
      n34 = global write "GVAIs.vi" "AIs"(w68) -> ()
      n35 = Array Size(array=w80) -> (size(s)=w79:i32[])
      n36 = local read "ECDSpeichern"() -> (w95:bool)
      n37 = property on="Methode" class="Ring (strict)"("Strings []"=w185) -> ()  [unwired: 2 in, 2 out]
      n38 = for {
        tunnel: w79 -> [w204] mode=indexing
        tunnel: [w201] -> w78 mode=indexing
        n39 = Initialize Array(FALSE, w204) -> (w202:bool[])
        n40 = Bundle(w202) -> (w201:cluster{bool[]})  [unwired: 1 in]
      }
      n41 = local read "HKSpeichern"() -> (w96:bool)
      n42 = Open/Create/Replace File(file path (use dialog)=path "c:/fromcriocmd.txt" ("Pfad MS-Datei CRIO"), operation (0:open)=T4."replace or create" ("Operation (0:Öffnen)")) -> (refnum out=w154:refnum<file>, error out=w153:errorcluster)  [unwired: 4 in, 1 out]
      n43 = Open/Create/Replace File(file path (use dialog)=path "c:/fromcriordy.txt" ("Dateipfad (Dialog verwenden)"), operation (0:open)=T4."replace or create" ("Operation (0:Öffnen)")) -> (refnum out=w148:refnum<file>, error out=w149:errorcluster)  [unwired: 4 in, 1 out]
      n44 = Write to Text File(file (use dialog)=w154, text="time=              \ncycle=   \ninfo=                                                                                                                                                      \nlength=   \ncmd=" ("Text0 MS-Datei"), error in=w153) -> (refnum out=w151:refnum<file>, error out=w150:errorcluster)  [unwired: 1 in, 1 out]
      n45 = case shown="True" w95 {
        tunnel: [w205 w214] -> w160
        tunnel: [w205 w213] -> w159
        tunnel: [w205 w212] -> w158
        tunnel: [w205 w211] -> w157
        tunnel: w109 -> [_ w210]
        tunnel: w108 -> [_ w209]
        tunnel: w107 -> [_ w208]
        tunnel: w106 -> [_ w207]
        tunnel: w97 -> [_ w206]
        frame False {
          w205 = refnum<k34> refnum ("tdms0")
        }
        frame True {
          n46 = call "TDMS0.vi"("Startmethode"=w206, "Dateiname"=w207, "Dateiordner"=w208) -> ("tdms1"=w211:refnum<k34>, "tdms0"=w212:refnum<k34>)
          n47 = call "TDMS0.vi"("Startmethode"=w206, "Dateiname"=w209, "Dateiordner"=w210) -> ("tdms1"=w213:refnum<k34>, "tdms0"=w214:refnum<k34>)
          n48 = global write "GVaktuelleTDMS.vi" "aktuelleTDMS-DateiECD1"(w214) -> ()
          n49 = global write "GVaktuelleTDMS.vi" "aktuelleTDMS-DateiECD2"(w212) -> ()
        }
      }
      n50 = global write "GVZwangs.vi" "ZwangsDIO!"(w78) -> ()
      n51 = global write "GVZwangs.vi" "ZwangsDIO?"(w78) -> ()
      n52 = Close File(refnum=w148, error in=w149) -> (path=w181:path)  [unwired: 1 out]
      n53 = Array Size(array=w71) -> (size(s)=w70:i32)
      n54 = case shown="True" w96 {
        tunnel: [w215 w220] -> w162
        tunnel: [w215 w219] -> w161
        tunnel: w111 -> [_ w218]
        tunnel: w110 -> [_ w217]
        tunnel: w97 -> [_ w216]
        frame False {
          w215 = refnum<k34> refnum ("tdms1")
        }
        frame True {
          n55 = call "TDMS0.vi"("Startmethode"=w216, "Dateiname"=w217, "Dateiordner"=w218) -> ("tdms1"=w219:refnum<k34>, "tdms0"=w220:refnum<k34>)
          n56 = global write "GVaktuelleTDMS.vi" "aktuelleTDMS-DateiHK"(w220) -> ()
        }
      }
      n57 = for {
        tunnel: w74 -> [w199] mode=indexing
        tunnel: [w196] -> w73 mode=indexing
        tunnel: [w194] -> w72 mode=indexing
        n58 = Initialize Array(0.0 ("Element"), w199) -> (w197:dbl[])
        n59 = Initialize Array(FALSE, w199) -> (w195:bool[])
        n60 = Bundle(w197) -> (w196:cluster{dbl[]})  [unwired: 1 in]
        n61 = Bundle(w195) -> (w194:cluster{bool[]})  [unwired: 1 in]
      }
      n62 = Close File(refnum=w151, error in=w150) -> (path=w145:path)  [unwired: 1 out]
      n63 = Initialize Array(FALSE, 6 ("Dimension")) -> (w75:bool[])
      n64 = Initialize Array(FALSE, w70) -> (w65:bool[])
      n65 = global write "GVZwangs.vi" "ZwangsFPGABoolesch?"(w75) -> ()
      n66 = global write "GVZwangs.vi" "ZwangsFPGABoolesch!"(w75) -> ()
      n67 = global write "GVZwangs.vi" "ZwangsLangsameH?"(w65) -> ()
      n68 = global write "GVZwangs.vi" "ZwangsLangsameH!"(w65) -> ()
      n69 = global write "GVZwangs.vi" "ZwangsHorst!"(w73) -> ()
      n70 = global write "GVZwangs.vi" "ZwangsHorst?"(w72) -> ()
      n71 = global write "GVHK1Hz.vi" "Mod1Mod2Mod3/AITrapsMachs1Hz"(w66) -> ()
      n72 = global write "GVHeizenLH.vi" "Heizen?LH"(w65) -> ()
      n73 = global write "GVECDs.vi" "ECD1Empfangen?"(w64) -> ()
      n74 = global write "GVECDs.vi" "ECD2Empfangen?"(w64) -> ()
      n75 = global write "GVECDs.vi" "ECD2MW"(w63) -> ()
      n76 = global write "GVECDs.vi" "ECD1MW"(w63) -> ()
      n77 = Build Array (concatenate)(w115, w114, w113, w112) -> (w53:string[])
      n78 = Build Array (concatenate)(w142, w141, w140, w139) -> (w192:string[])
      n79 = Build Array (concatenate)(w130, w129, w128, w127) -> (w190:string[])
      n80 = Initialize Array(0.0 ("Element"), 6 ("Dimension")) -> (w60:dbl[])
      n81 = global write "GVZeitenZyklen.vi" "Big Ben, Methodenzeit, Zykluszeit0, Zykluszeit1, Zykluszeit2A, Zykluszeit2B"(w60) -> ()
      n82 = Build Array (concatenate)(w138, w137, w136, w135) -> (w191:string[])
      n83 = Add Array Elements(numeric array=w74) -> (sum=w176:i32)
      n84 = Build Array (concatenate)(w134, w133, w132, w131) -> (w184:dbl[])
      n85 = Build Array (concatenate)(w54, w53) -> (w52:string[])
      n86 = Initialize Array(0, 4 ("Dimension")) -> (w57:i32[])
      n87 = Split 1D Array(array=w187, index=2 ("Index")) -> (second subarray=w179:string[])  [unwired: 1 out]
      n88 = property on="Zeitachse1" class="Ring (strict)"("Strings []"=w179) -> ()  [unwired: 2 in, 2 out]
      n89 = property on="Zeitachse2" class="Ring (strict)"("Strings []"=w179) -> ()  [unwired: 2 in, 2 out]
      n90 = global write "GVZeitenZyklen.vi" "ZyklusNummernGesamt"(w57) -> ()
      n91 = global write "GVZeitenZyklen.vi" "ZyklusNummern"(w57) -> ()
      n92 = global write "GVVentilposition.vi" "Ventilposition"(1 ("Ventilposition")) -> ()
      n93 = Build Array (concatenate)(w43, w54, w53) -> (w50:string[])
      n94 = property on="dargestellte Größe 3" class="Ring (strict)"("Strings []"=w52) -> ()  [unwired: 2 in, 2 out]
      n95 = Index Array(array=w123, index (col)=2 ("Deaktivierter Index (Spalte)")) -> (element=w172:dbl[])  [unwired: 1 in]
      n96 = Index Array(array=w123, index (col)=1 ("Deaktivierter Index (Spalte)")) -> (element=w171:dbl[])  [unwired: 1 in]
      n97 = Index Array(array=w123, index (col)=0 ("Deaktivierter Index (Spalte)")) -> (element=w170:dbl[])  [unwired: 1 in]
      n98 = call "AIKoeffSortieren.vi"("Modul3/AI koeff"=w124, "Modul2/AI koeff"=w125, "Modul1/AI koeff"=w126) -> ("P0"=w166:dbl[], "P1"=w167:dbl[], "P2"=w168:dbl[])
      n99 = Build Cluster Array(w84, w83, w82, w81) -> (w183:cluster{"DIOsMod2BNr":i32[]}[])
      n100 = for {
        tunnel: w183 -> [w224] mode=indexing
        tunnel: [w225] -> w182 mode=indexing
        n101 = Unbundle(w224) -> ("DIOsMod2BNr"=w223:i32[])
        n102 = Array Size(array=w223) -> (size(s)=w225:i32)
      }
      n103 = property on="dargestellte Größe 1" class="Ring (strict)"("Strings []"=w50) -> ()  [unwired: 2 in, 2 out]
      n104 = property on="dargestellte Größe 2" class="Ring (strict)"("Strings []"=w50) -> ()  [unwired: 2 in, 2 out]
      n105 = Bundle("DIOsMod0Name"=w119, "DIOsMod1Name"=w118, "DIOsMod2AName"=w117, "DIOsMod2BName"=w116, "HorstMod0Name"=w115, "HorstMod1Name"=w114, "HorstMod2AName"=w113, "HorstMod2BName"=w112, "NamenLangsameHeizungen"=w105) -> (w180:T11)  [unwired: 1 in]
      n106 = Build Array (concatenate)(string[] ["Datei Nr.", "Zyklusnr. Mod0", "Zyklusnr. Mod1", "Zyklusnr. Mod2A", "Zyklusnr. Mod2B"], w187, w43, w54, w53, "Probenvolumen1", "Probenvolumen2") -> (w189:string[])
      n107 = Array Subset(array=w43, index=0 ("Index"), length=32 ("Länge")) -> (→"AIs1":string[])
      n108 = Array Subset(array=w43, index=32 ("Index"), length=32 ("Länge")) -> (→"AIs2":string[])
      n109 = Array Subset(array=w43, index=64 ("Index"), length=32 ("Länge")) -> (→"AIs3":string[])
      n110 = Bundle("Dateiordner Housekeeping"=w111, "DateiordnerECD1"=w109, "DateiordnerECD2"=w107, "Dateiname Housekeeping"=w110, "DateinameECD1"=w108, "DateinameECD2"=w106, "tdms0"=w162, "tdms1"=w161, "tdms0"=w160, "tdms1"=w159, "tdms0"=w158, "tdms1"=w157) -> (w163:T12)  [unwired: 1 in]
      n111 = Array Size(array=w105) -> (size(s)=w104:i32)
    }
    frame #1 {
      w226 = dbl[] [-1.0]
      w301 = 0
      w276 = 0 ("Zyklusnummer1")
      n112 = while {
        shift-right: ["Methode"] -> _
        shift-left: w330 -> [w1190]
        stop <- w1192 stop-if-true
        n113 = call "Bis zum nächsten Vielfachen warten7"("Count(mSec)"=u32 1000) -> ()  [unwired: 1 out]
        n114 = Not Equal?(x=w1190, y="Methode") -> (x != y?=w1188:bool)
        n115 = global write "GVMethodenwechsel.vi" "Methodenwechsel?"(w1188) -> ()
        n116 = global read "gvbooleschRT.vi" "global stop RT"() -> (w1192:bool)
      }
      n117 = Add Array Elements(numeric array=w248) -> (sum=w247:i32)
      n118 = flat-sequence {
        frame #0 {
          n119 = call "Warten5"("Count(mSec)"=u32 1000) -> ()  [unwired: 1 out]
        }
        frame #1 {
          n120 = case shown="True" "Licor" {
            frame False {
            }
            frame True {
              w362 = i16 128 items=["Unknown"=-1, "RS485/Wire4"=0, "RS485/Wire2-EchoDTR"=1, "RS485/Wire2-CtrlDTR"=2, "RS485/Wire2-Auto"=3, "RS232/DTE"=128, "RS232/DCE"=129, "RS232/AUTO"=130] ("Serial Settings:Wire Mode")
              n121 = call-poly "VISA Configure Serial Port"("VISA resource name"=refnum<visa-resource-name> "ASRL1::INSTR") -> ("VISA resource name out"=w361:refnum<visa-resource-name>)  [unwired: 13 in, 1 out]
              n122 = property class="Instr"(reference=w361, "Wire Mode"=w362) -> (reference out=w360:refnum<visa-resource-name>)  [unwired: 1 in, 1 out]
              n123 = VISA Flush I/O Buffer(VISA resource name=w360) -> (VISA resource name out=w359:refnum<visa-resource-name>)  [unwired: 2 in, 1 out]
              n124 = while {
                tunnel: w359 -> [w371]
                shift-right: [w373] -> _
                shift-left: "xxx" -> [w375]
                tunnel: [w367] -> w364
                stop <- w376 stop-if-true
                n125 = property class="Instr"(reference=w371) -> (reference out=w370:refnum<visa-resource-name>, "Serial Settings:Number of Bytes at Serial Port"=w369:u32)  [unwired: 1 in, 1 out]
                n126 = call "Warten4"("Count(mSec)"=u32 500) -> ()  [unwired: 1 out]
                n127 = VISA Read(VISA resource name=w370, byte count=w369) -> (VISA resource name out=w368:refnum<visa-resource-name>, read buffer=w374:string)  [unwired: 1 in, 2 out]
                n128 = global read "gvbooleschRT.vi" "global stop RT"() -> (w376:bool)
                n129 = Concatenate Strings(w375, w374) -> (w373:string)
                "vomLicor" <- w373
                n130 = case shown="False" "senden" {
                  tunnel: w368 -> [w377 w379]
                  tunnel: [w377 w378] -> w367
                  frame False {
                  }
                  frame True {
                    n131 = Concatenate Strings("Schreibpuffer", "\n") -> (w380:string)
                    n132 = VISA Write(VISA resource name=w379, write buffer=w380) -> (VISA resource name out=w378:refnum<visa-resource-name>)  [unwired: 1 in, 2 out]
                  }
                }
              }
              n133 = VISA Close(VISA resource name=w364) -> ()  [unwired: 1 in, 1 out]
            }
          }
        }
      }
      n134 = Array Size(array=w258) -> (size(s)=w279:i32)
      n135 = Index Array(array=w243, index=w241) -> (element=w242:T13)
      n136 = while {
        stop <- w1176 stop-if-true
        w1170 = 10.0
        n137 = global read "GVTrapsMachs.vi" "Traps/Machs"() -> (w1166:dbl[])
        n138 = global read "GVAIs.vi" "AIs"() -> (w1167:dbl[])
        n139 = call "Warten2"("Count(mSec)"=u32 1000) -> ()  [unwired: 1 out]
        n140 = for {
          N: 9 -> [_]
          shift-right: [w1179] -> w1173
          shift-left: w1167 -> [w1180]
          shift-right: [w1177] -> w1171
          shift-left: w1166 -> [w1178]
          n141 = flat-sequence {
            tunnel: w1180 -> [w1187]
            tunnel: [w1186] -> w1179
            tunnel: w1178 -> [w1185]
            tunnel: [w1184] -> w1177
            frame #0 {
              n142 = call "Warten28"("Count(mSec)"=u32 100) -> ()  [unwired: 1 out]
            }
            frame #1 {
              n143 = global read "GVTrapsMachs.vi" "Traps/Machs"() -> (w1182:dbl[])
              n144 = global read "GVAIs.vi" "AIs"() -> (w1183:dbl[])
              n145 = Add(x=w1187, y=w1183) -> (x+y=w1186:dbl[])
              n146 = Add(x=w1182, y=w1185) -> (x+y=w1184:dbl[])
            }
          }
        }
        n147 = Divide(x=w1173, y=w1170) -> (x/y=w1172:dbl[])
        n148 = Divide(x=w1171, y=w1170) -> (x/y=w1169:dbl[])
        n149 = Build Array (concatenate)(w1172, w1169) -> (w1168:dbl[])
        n150 = global write "GVHK1Hz.vi" "Mod1Mod2Mod3/AITrapsMachs1Hz"(w1168) -> ()
        n151 = global read "gvbooleschRT.vi" "global stop RT"() -> (w1176:bool)
      }
      n152 = while {
        tunnel: w254 -> [w684]
        tunnel: w323 -> [w683]
        tunnel: w322 -> [w682]
        tunnel: w321 -> [w681]
        stop <- w685 stop-if-true
        n153 = call "AIsFIFORT.vi"("P0"=w681, "P1"=w682, "P2"=w683, "FPGA VI Reference In"=w684) -> ()  [unwired: 1 in]
        n154 = global read "gvbooleschRT.vi" "global stop RT"() -> (w685:bool)
      }
      n155 = Initialize Array(cluster{"output high":dbl, "output low":dbl} {"output high"=99999.0, "output low"=0.0} ("output range"), w279) -> (w259:cluster{"output high":dbl, "output low":dbl}[])
      n156 = while {
        tunnel: w254 -> [w686]
        tunnel: w326 -> [w690]
        tunnel: w325 -> [w688]
        tunnel: w324 -> [w687]
        stop <- w691 stop-if-true
        n157 = call "TrapsMachMitteln.vi"("Traps/MachKoeff0"=w687, "Traps/MachKoeff1"=w688, "Traps/MachKoeff2"=w690, "FPGA VI Reference In"=w686) -> ()  [unwired: 1 in]
        n158 = global read "gvbooleschRT.vi" "global stop RT"() -> (w691:bool)
        n159 = call "Bis zum nächsten Vielfachen warten16"("Count(mSec)"=u32 100) -> ()  [unwired: 1 out]
      }
      n160 = Initialize Array(-1 ("Element"), 4 ("Dimension")) -> (w250:i32[])
      n161 = while {
        tunnel: w329 -> [w797]
        shift-right: [w796] -> _
        shift-left: w243 -> [w774]
        tunnel: w259 -> [w795]
        tunnel: w258 -> [w794]
        tunnel: w254 -> [w793]
        tunnel: w257 -> [w792]
        tunnel: w256 -> [w791]
        shift-right: [w783] -> _
        shift-left: 0 -> [w790]
        tunnel: w254 -> [w789]
        tunnel: w253 -> [w788]
        shift-right: [w782] -> _
        shift-left: 0.0 -> [w787]
        shift-right: [w781] -> _
        shift-left: -1 -> [w786]
        shift-right: [w780] -> _
        shift-left: w250 -> [w785]
        tunnel: w249 -> [w775]
        tunnel: w248 -> [w776]
        tunnel: w247 -> [w777]
        tunnel: w246 -> [w778]
        tunnel: w245 -> [w779]
        tunnel: w244 -> [w784]
        shift-right: [w695] -> _
        shift-left: w242 -> [w694]
        i -> [w698]
        stop <- w798 stop-if-true
        w740 = FALSE
        w739 = 0.0
        w741 = 0  # ZeilennummerMPV
        w745 = cluster{dbl[], dbl[]} {[], []}
        w755 = dbl[] []
        w759 = 0  # ZeileMach2
        w760 = 0  # ZeileMach1
        w761 = 0  # ZeileFPGAFixp
        w762 = 0  # ZeileFPGAPID
        w763 = 0  # ZeileFPGABoolesch
        w764 = i32[] [0, 0, 0, 0]  # ZeilennummernHorst
        w765 = i32[] [0, 0, 0, 0]  # ZeilennummernDIOs
        n162 = local read "Methode"() -> (w697:i32)
        n163 = Index Array(array=w774, index=w697) -> (element=w696:T13)
        n164 = Unbundle(w694) -> ("Zykluslängen [s]"=w738:dbl[], "ZeitpktDIOsMod0"=w737:dbl[], "ZeitpktDIOsMod1"=w736:dbl[], "ZeitpktDIOsMod2A"=w735:dbl[], "ZeitpktDIOsMod2B"=w734:dbl[], "DIOsSPMod0"=w733:bool[][], "DIOsSPMod1"=w732:bool[][], "DIOsSPMod2A"=w731:bool[][], "DIOsSPMod2B"=w730:bool[][], "Mod0HorstZeitpkt"=w729:dbl[], "Mod1HorstZeitpkt"=w728:dbl[], "Mod2AHorstZeitpkt"=w727:dbl[], "Mod2BHorstZeitpkt"=w726:dbl[], "HorstSPMod0"=w725:dbl[][], "HorstSPMod1"=w724:dbl[][], "HorstSPMod2A"=w723:dbl[][], "HorstSPMod2B"=w722:dbl[][], "LangsameHeizungenSP"=w721:dbl[], "LHHeizen?"=w720:bool[], "ZPktFPGABoolesch"=w719:dbl[], "FPGABoolesch"=w718:bool[][], "ZeitpktFPGAPID"=w717:dbl[], "FPGAPID"=w716:T14, "ZeitpktFPGAFixp"=w715:dbl[], "FPGAFixp"=w714:fxp<+/-,16,4>[][], "ZeitpktMach1"=w713:dbl[], "TempMach1"=w712:dbl[], "ZeitpktMach2"=w711:dbl[], "TempMach2"=w710:dbl[], "PIDs für \"träge\" Heizungen"=w709:T15, "Zwangsbedingungen"=w708:dbl[][], "Dateien fürs MS schicken?"=w707:bool, "ZeitpunkteMPV"=w706:dbl[], "SPMPV"=w705:i32[], "ZeitpktMSa"=w704:dbl, "ZeitpktMSb"=w703:dbl, "Int.Start1"=w702:dbl, "Int.Stop1"=w701:dbl, "Int.Start2"=w700:dbl, "Int.Stop2"=w699:dbl)  [unwired: 1 out]
        "Zykluslängen [s]" <- w738
        n165 = Add(x=w785, y=1) -> (x+y=w749:i32[])
        n166 = Add(x=w786, y=1) -> (x+y=w771:i32)
        n167 = global read "GVaktuelleTDMS.vi" "aktuelleTDMS-DateiECD1"() -> (w747:refnum<k34>)
        n168 = global read "GVZwangs.vi" "ZwangsFPGABoolesch?"() -> (w752:bool[])
        n169 = global read "GVZeitenZyklen.vi" "ZyklusNummern"() -> (w748:i32[])
        n170 = global read "GVZwangs.vi" "ZwangsHorst?"() -> (w754:cluster{bool[]}[])
        n171 = global read "GVZwangs.vi" "ZwangsDIO?"() -> (w753:cluster{bool[]}[])
        n172 = while {
          tunnel: w776 -> [w950]
          tunnel: w779 -> [w948]
          tunnel: w778 -> [w947]
          tunnel: w775 -> [w949]
          tunnel: w777 -> [w946]
          tunnel: w708 -> [w938]
          stop <- w940 stop-if-true
          n173 = local read "Methode"() -> (w945:i32)
          n174 = global read "gvbooleschRT.vi" "global stop RT"() -> (w943:bool)
          n175 = case shown="True" "global stop RT" {
            frame False {
            }
            frame True {
              n176 = global write "gvbooleschRT.vi" "global stop RT"(TRUE ("global stop RT")) -> ()
            }
          }
          n177 = call "ZwangsbedingungenGV.vi"("AnzahlHorst"=w948, "AnzahlHorst/Modul"=w949, "AnzahlLH"=w947, "AnzahlDIOs/Modul"=w950, "AnzahlDIOs"=w946, "Zwangsbedingungen"=w938, "Methodennummer"=w945) -> ("Methodennummer"=w944:i32)  [unwired: 4 in]
          n178 = local read "veränderte Methode benutzen"() -> (w941:bool)
          n179 = global read "GVMethodenwechsel.vi" "Methodenwechsel?"() -> (w942:bool)
          n180 = local write "Methode"(w944) -> ()
          n181 = Compound Arithmetic op=OR(w943, w942, w941) -> (w940:bool)
          n182 = call "Bis zum nächsten Vielfachen warten10"("Count(mSec)"=u32 1000) -> ()  [unwired: 1 out]
        }
        n183 = while {
          tunnel: w794 -> [w861]
          tunnel: w795 -> [w862]
          tunnel: w793 -> [w858]
          tunnel: w721 -> [w852]
          tunnel: w709 -> [w851]
          stop <- w847 stop-if-true
          n184 = global read "GVAIs.vi" "AIs"() -> (w853:dbl[])
          n185 = call "Bis zum nächsten Vielfachen warten12"("Count(mSec)"=u32 100) -> ()  [unwired: 1 out]
          n186 = for {
            tunnel: w853 -> [w937]
            tunnel: w861 -> [w936] mode=indexing
            tunnel: [w935] -> w860 mode=indexing
            n187 = Index Array(array=w937, index=w936) -> (element=w935:dbl)
          }
          n188 = global read "gvbooleschRT.vi" "global stop RT"() -> (w850:bool)
          n189 = local read "veränderte Methode benutzen"() -> (w848:bool)
          n190 = global read "GVMethodenwechsel.vi" "Methodenwechsel?"() -> (w849:bool)
          n191 = call-poly <vilib>:"PID.vi"("output range"=w862, "PID gains"=w851, "process variable"=w860, "setpoint"=w852) -> ("output"=w859:dbl[])  [unwired: 6 in, 1 out]
          n192 = global read "GVHeizenLH.vi" "Heizen?LH"() -> (w854:bool[])
          n193 = Compound Arithmetic op=OR(w850, w849, w848) -> (w847:bool)
          n194 = To Unsigned Long Integer(number=w859) -> (unsigned 32bit integer=w856:u32[])
          n195 = Array To Cluster(array=w854) -> (cluster=w857:T16)
          n196 = Array To Cluster(array=w856) -> (cluster=w855:T17)
          n197 = xnode "Read/Write Control"("FPGA VI Reference In"=w858, "LHHeizen?"=w857, "LHPulse(us)"=w855) -> ()  [unwired: 1 in, 2 out]
        }
        n198 = while {
          tunnel: w797 -> [w1142]
          shift-right: [w1133] -> _
          shift-left: w696 -> [w1141]
          tunnel: w697 -> [w1139]
          shift-right: [w1131] -> w796
          shift-left: w774 -> [w1140]
          tunnel: [w1132] -> w695
          stop <- w1135 stop-if-true
          n199 = global read "GVMethodenwechsel.vi" "Methodenwechsel?"() -> (w1137:bool)
          n200 = global read "gvbooleschRT.vi" "global stop RT"() -> (w1136:bool)
          n201 = case shown="True" "Methode verändern" {
            tunnel: w1142 -> [_ w1164]
            tunnel: w1141 -> [w1161 w1163]
            tunnel: [w1161 w1162] -> w1133
            frame False {
            }
            frame True {
              n202 = call "methodeändern.vi"("Methode"=w1163, "Namen"=w1164) -> ("Methode"=w1162:T13)  [unwired: 1 in]
              n203 = property on="Methode verändern" class="Bool (strict)"("Value"=FALSE ("Methode verändern")) -> ()  [unwired: 2 in, 2 out]
            }
          }
          n204 = Compound Arithmetic op=OR(w1137, w1136, "veränderte Methode benutzen") -> (w1135:bool)
          n205 = case shown="True" "Methode speichern" {
            tunnel: w1133 -> [_ w1158]
            tunnel: w1140 -> [w1151 w1160]
            tunnel: w1139 -> [_ w1159]
            tunnel: [w1151 w1153] -> w1131
            frame False {
            }
            frame True {
              n206 = Replace Array Subset(array=w1160, new element=w1158, index=w1159) -> (w1153:T2)
              n207 = property on="Methode speichern" class="Bool (strict)"("Value"=FALSE ("Methode speichern")) -> ()  [unwired: 2 in, 2 out]
              n208 = Open/Create/Replace File(file path (use dialog)=path "c:/methoden.per" ("Dateipfad (Dialog verwenden)"), operation (0:open)=T4."replace" ("Operation (0:Öffnen)")) -> (refnum out=w1155:refnum<file>)  [unwired: 4 in, 2 out]
              n209 = Write to Binary File(file (use dialog)=w1155, data=w1153) -> (refnum out=w1152:refnum<file>)  [unwired: 4 in, 2 out]
              n210 = Close File(refnum=w1152) -> ()  [unwired: 1 in, 2 out]
            }
          }
          n211 = case shown="False" "veränderte Methode benutzen" {
            tunnel: w1133 -> [_ w1148]
            tunnel: [w1145 w1148] -> w1132
            tunnel: w1131 -> [w1147 _]
            frame False {
              n212 = local read "Methode"() -> (w1146:i32)
              n213 = Index Array(array=w1147, index=w1146) -> (element=w1145:T13)
            }
            frame True {
              n214 = flat-sequence {
                frame #0 {
                  n215 = call "Warten"("Count(mSec)"=u32 1100) -> ()  [unwired: 1 out]
                }
                frame #1 {
                  n216 = property on="veränderte Methode benutzen" class="Bool (strict)"("Value"=FALSE ("Methode verändern")) -> ()  [unwired: 2 in, 2 out]
                }
              }
            }
          }
          n217 = call "Bis zum nächsten Vielfachen warten8"("Count(mSec)"=u32 500) -> ()  [unwired: 1 out]
        }
        n218 = Build Cluster Array(w733, w732, w731, w730) -> (w769:cluster{"DIOsSPMod2B":bool[][]}[])
        n219 = Build Cluster Array(w725, w724, w723, w722) -> (w767:cluster{"HorstSPMod2B":dbl[][]}[])
        n220 = Bundle(w755, w755, w755, w755) -> (w756:cluster{dbl[], dbl[], dbl[], dbl[]})  [unwired: 1 in]
        n221 = Build Cluster Array(w737, w736, w735, w734) -> (w770:cluster{"ZeitpktDIOsMod2B":dbl[]}[])
        n222 = Build Cluster Array(w729, w728, w727, w726) -> (w768:cluster{"Mod2BHorstZeitpkt":dbl[]}[])
        n223 = Equal?(x=w698, y=0) -> (x = y?=w772:bool)
        n224 = while {
          shift-right: [w811] -> _
          shift-left: w740 -> [w815]
          shift-right: [w810] -> _
          shift-left: w739 -> [w814]
          shift-right: [w809] -> _
          shift-left: w740 -> [w813]
          shift-right: [w808] -> _
          shift-left: w739 -> [w812]
          tunnel: w784 -> [w807]
          tunnel: w702 -> [w802]
          tunnel: w701 -> [w801]
          tunnel: w700 -> [w800]
          tunnel: w699 -> [w799]
          stop <- w804 stop-if-true
          n225 = call "Integrieren.vi"("Integrieren1"=w815, "Integral1"=w814, "Integrieren2"=w813, "Integral2"=w812, "Int.Start1"=w802, "Int.Stop1"=w801, "Int.Start2"=w800, "HorstProbenflußNr."=w807, "Int.Stop2"=w799) -> ("Integrieren1"=w811:bool, "Integral1"=w810:dbl, "Integrieren2"=w809:bool, "Integral2"=w808:dbl)  [unwired: 7 in]
          n226 = global read "gvbooleschRT.vi" "global stop RT"() -> (w806:bool)
          n227 = local read "veränderte Methode benutzen"() -> (w803:bool)
          n228 = global read "GVMethodenwechsel.vi" "Methodenwechsel?"() -> (w805:bool)
          n229 = Compound Arithmetic op=OR(w806, w805, w803) -> (w804:bool)
          n230 = call "Bis zum nächsten Vielfachen warten9"("Count(mSec)"=u32 100) -> ()  [unwired: 1 out]
        }
        n231 = Bundle(w770, w769, w768, w767, "LHHeizen?"=w720, "ZPktFPGABoolesch"=w719, "FPGABoolesch"=w718, "ZeitpktFPGAPID"=w717, "FPGAPID"=w716, "ZeitpktFPGAFixp"=w715, "FPGAFixp"=w714, "ZeitpktMach1"=w713, "TempMach1"=w712, "ZeitpktMach2"=w711, "TempMach2"=w710, "ZeitpunkteMPV"=w706, "SPMPV"=w705) -> (w766:T18)  [unwired: 1 in]
        n232 = Bundle("ZyklusNummern"=w748, "ZeilennummernDIOs"=w765, "ZwangsDIO?"=w753, "ZeilennummernHorst"=w764, "ZwangsHorst?"=w754, "ZeileFPGABoolesch"=w763, "ZwangsFPGABoolesch?"=w752, "ZeileFPGAPID"=w762, "ZeileFPGAFixp"=w761, "ZeileMach1"=w760, "ZeileMach2"=w759, "ZeilennummerMPV"=w741) -> (w758:T19)  [unwired: 1 in]
        n233 = while "ZyklusSteuerung" {
          tunnel: w788 -> [w1059]
          tunnel: w789 -> [w1057]
          shift-right: [w1055] -> _
          shift-left: w758 -> [w1056]
          tunnel: w766 -> [w1058]
          stop <- w1051 stop-if-true
          n234 = call "ZyklussteuerungGV.vi"("Zeitpunkte/SPs"=w1058, "DIOsNummern"=w1059, "Schieberegister"=w1056, "FPGA VI Reference In"=w1057) -> ("Schieberegister"=w1055:T20)  [unwired: 2 in]
          n235 = global read "gvbooleschRT.vi" "global stop RT"() -> (w1053:bool)
          n236 = local read "veränderte Methode benutzen"() -> (w1052:bool)
          n237 = global read "GVMethodenwechsel.vi" "Methodenwechsel?"() -> (w1054:bool)
          n238 = Compound Arithmetic op=OR(w1054, w1053, w1052) -> (w1051:bool)
          n239 = call "Bis zum nächsten Vielfachen warten11"("Count(mSec)"=u32 100) -> ()  [unwired: 1 out]
        }
        n240 = while {
          shift-right: [w999] -> _
          shift-left: w756 -> [w1006]
          shift-right: [w998] -> _
          shift-left: w756 -> [w1005]
          shift-right: [w996] -> _
          shift-left: T10 {"Zyklus1"=0, "Zeitachse1"=0, "dargestellte Größe 1"=0, "Zyklus2"=0, "Zeitachse2"=0, "dargestellte Größe 2"=0} ("AnzeigeEinstellungen") -> [w1004]
          tunnel: w738 -> [w974]
          shift-right: [w970] -> _
          shift-left: w747 -> [w969]
          shift-right: [w965] -> _
          shift-left: w745 -> [w967]
          shift-right: [w954] -> _
          shift-left: w745 -> [w966]
          shift-right: ["Detektor"] -> _
          shift-left: 0 ("Detektor") -> [w963]
          stop <- w1010 stop-if-true
          w975 = 0.0 ("X-Achse.Bereich:Minimum")
          n241 = case shown="0, Default" "Detektor" {
            tunnel: [w1030 w1042] -> w965
            tunnel: w974 -> [w1029 w1044]
            tunnel: "Detektor" -> [w1024 w1038]
            tunnel: [w1028 w1043] -> w972
            tunnel: [w1027 w1041] -> w970
            frame 0, Default {
              n242 = Increment(x=w1024) -> (x+1=w1025:i32)
              n243 = Increment(x=w1025) -> (x+1=w1023:i32)
              n244 = Index Array(array=w1029, index=w1023) -> (element=w1028:dbl)
              n245 = global read "GVaktuelleTDMS.vi" "aktuelleTDMS-DateiECD1"() -> (w1027:refnum<k34>)
              n246 = global read "GVChroms.vi" "ECD1Chrom"() -> (w1026:dbl[])
              n247 = Array Size(array=w1026) -> (size(s)=w1032:i32)
              n248 = for {
                N: w1032 -> [_]
                tunnel: [w1033] -> w1031 mode=indexing
                i -> [w1036]
                n249 = To Double Precision Float(number=w1036) -> (double precision float=w1035:dbl)
                n250 = Divide(x=w1035, y=10.0) -> (x/y=w1033:dbl)
              }
              n251 = Bundle(w1031, "ECD1Chrom"=w1026) -> (w1030:cluster{dbl[], "ECD1Chrom":dbl[]})  [unwired: 1 in]
            }
            frame 1 {
              n252 = Increment(x=w1038) -> (x+1=w1039:i32)
              n253 = Increment(x=w1039) -> (x+1=w1037:i32)
              n254 = Index Array(array=w1044, index=w1037) -> (element=w1043:dbl)
              n255 = global read "GVaktuelleTDMS.vi" "aktuelleTDMS-DateiECD2"() -> (w1041:refnum<k34>)
              n256 = global read "GVChroms.vi" "ECD2Chrom"() -> (w1040:dbl[])
              n257 = Array Size(array=w1040) -> (size(s)=w1046:i32)
              n258 = for {
                N: w1046 -> [_]
                tunnel: [w1047] -> w1045 mode=indexing
                i -> [w1050]
                n259 = To Double Precision Float(number=w1050) -> (double precision float=w1049:dbl)
                n260 = Divide(x=w1049, y=10.0) -> (x/y=w1047:dbl)
              }
              n261 = Bundle(w1045, "ECD2Chrom"=w1040) -> (w1042:cluster{dbl[], "ECD2Chrom":dbl[]})  [unwired: 1 in]
            }
          }
          n262 = case shown="True" "Tabellarische Darstellung" {
            frame False {
            }
            frame True {
              n263 = global read "GVHK1Hz.vi" "Mod1Mod2Mod3/AITrapsMachs1Hz"() -> (w1016:dbl[])
              n264 = Array Subset(array=w1016, index=32 ("Index"), length=32 ("Länge")) -> (→"AIs2":dbl[])
              n265 = Array Subset(array=w1016, index=64 ("Index"), length=32 ("Länge")) -> (→"AIs3":dbl[])
              n266 = Array Subset(array=w1016, index=0 ("Index"), length=32 ("Länge")) -> (→"AIs1":dbl[])
            }
          }
          n267 = global read "GVZeitenZyklen.vi" "Big Ben, Methodenzeit, Zykluszeit0, Zykluszeit1, Zykluszeit2A, Zykluszeit2B"() -> (w957:dbl[])
          n268 = global read "GVMethodenwechsel.vi" "Methodenwechsel?"() -> (w1008:bool)
          n269 = local read "veränderte Methode benutzen"() -> (w1007:bool)
          n270 = global read "gvbooleschRT.vi" "global stop RT"() -> (w1009:bool)
          n271 = global read "GVZeitenZyklen.vi" "ZyklusNummern"() -> (w977:i32[])
          "ZyklusNummern" <- w977
          n272 = Or(x=w1008, y=w1009) -> (x .or. y?=w1011:bool)
          n273 = To Long Integer(number=w957) -> (32bit integer=→"Big Ben, Methodenzeit, Zykluszeit0, Zykluszeit1, Zykluszeit2A, Zykluszeit2B":i32[])
          n274 = Or(x=w1011, y=w1007) -> (x .or. y?=w1010:bool)
          n275 = Subtract(x="HK1YMax", y="HK1YMin") -> (x-y=w990:dbl)
          n276 = Subtract(x="HK2YMax", y="HK2YMin") -> (x-y=w985:dbl)
          n277 = call "AnzeigeGV.vi"("veränderte Methode benutzen"=w1007, "Zykluslängen [s]"=w974, "Cluster1"=w1006, "Big Ben, Methodenzeit, Zykluszeit0, Zykluszeit1, Zykluszeit2A, Zykluszeit2B"=w957, "Zyklusnummern 0, 1, 2A, 2B"=w977, "Cluster2"=w1005, "AnzeigeEinstellungen"=w1004, "dargestellte Größe 1"="dargestellte Größe 1", "Zeitachse1"="Zeitachse1", "dargestellte Größe 2"="dargestellte Größe 2", "Zeitachse2"="Zeitachse2") -> ("Anzeige2"=→"Housekeeping2":cluster{dbl[], dbl[]}, "Cluster1"=w999:cluster{dbl[], dbl[], dbl[], dbl[]}, "x1Inkr"=w994:dbl, "Cluster2"=w998:cluster{dbl[], dbl[], dbl[], dbl[]}, "Anzeige1"=→"Housekeeping1":cluster{dbl[], dbl[]}, "AnzeigeEinstellungen"=w996:T10, "x2Max"=w958:dbl, "x2Inkr"=w993:dbl, "x1Max"=w959:dbl)  [unwired: 8 in]
          n278 = Divide(x=w990, y=10.0) -> (x/y=w988:dbl)
          n279 = Divide(x=w985, y=10.0) -> (x/y=w983:dbl)
          n280 = property on="Housekeeping1" class="XYGraph (strict)"("XScale.Minimum"=w975, "XScale.Maximum"=w959, "XScale.Increment"=w994, "YScale.Minimum"="HK1YMin", "YScale.Maximum"="HK1YMax", "YScale.Increment"=w988) -> ()  [unwired: 2 in, 2 out]
          n281 = property on="Housekeeping2" class="XYGraph (strict)"("XScale.Minimum"=w975, "XScale.Maximum"=w958, "XScale.Increment"=w993, "YScale.Minimum"="HK2YMin", "YScale.Maximum"="HK2YMax", "YScale.Increment"=w983) -> ()  [unwired: 2 in, 2 out]
          n282 = Subtract(x="DetYMax", y="DetYMin") -> (x-y=w980:dbl)
          n283 = global read "GVZeitenZyklen.vi" "ZyklusNummernGesamt"() -> (→"ZyklusNummernGesamt":i32[])
          n284 = Equal?(x=w970, y=w969) -> (x = y?=w968:bool)
          n285 = Divide(x=w972, y=20.0) -> (x/y=w973:dbl)
          n286 = Divide(x=w980, y=20.0) -> (x/y=w978:dbl)
          n287 = Equal?(x="Detektor", y=w963) -> (x = y?=w962:bool)
          n288 = Select(t=w966, s=w968, f=w967) -> (s? t:f=w961:cluster{dbl[], dbl[]})
          n289 = property on="Detektor" class="XYGraph (strict)"("XScale.Minimum"=w975, "XScale.Maximum"=w972, "XScale.Increment"=w973, "YScale.Minimum"="DetYMin", "YScale.Maximum"="DetYMax", "YScale.Increment"=w978) -> ()  [unwired: 2 in, 2 out]
          n290 = Select(t=w961, s=w962, f=cluster{dbl[], dbl[]} {[], []} ("s? t:f")) -> (s? t:f=w954:cluster{dbl[], dbl[]})
          n291 = Build Array(w965, w954) -> (→"Detektor":cluster{dbl[], "ECD2Chrom":dbl[]}[])
          n292 = call "Bis zum nächsten Vielfachen warten14"("Count(mSec)"=u32 1000) -> ()  [unwired: 1 out]
        }
        n293 = global read "GVZeitenZyklen.vi" "Big Ben, Methodenzeit, Zykluszeit0, Zykluszeit1, Zykluszeit2A, Zykluszeit2B"() -> (w744:dbl[])
        n294 = while "Zeit" {
          tunnel: w772 -> [w1080]
          tunnel: [w1075] -> w782
          tunnel: w787 -> [w1079]
          tunnel: [w1069] -> w781
          tunnel: w771 -> [w1070]
          tunnel: w738 -> [w1077]
          tunnel: w749 -> [w1064]
          tunnel: [w1061] -> w780
          i -> [w1083]
          stop <- w1066 stop-if-true
          n295 = Equal?(x=w1083, y=0) -> (x = y?=w1081:bool)
          n296 = And(x=w1080, y=w1081) -> (x .and. y?=w1085:bool)
          n297 = xnode "Elapsed Timer"("reset"=w1085) -> ("elapsed time (ms)"=w1088:i32)  [unwired: 2 in, 1 out]
          n298 = global read "gvbooleschRT.vi" "global stop RT"() -> (w1078:bool)
          n299 = global read "GVMethodenwechsel.vi" "Methodenwechsel?"() -> (w1065:bool)
          n300 = local read "veränderte Methode benutzen"() -> (w1068:bool)
          n301 = To Double Precision Float(number=w1088) -> (double precision float=w1087:dbl)
          n302 = Or(x=w1065, y=w1078) -> (x .or. y?=w1067:bool)
          n303 = Divide(x=w1087, y=1000.0) -> (x/y=w1075:dbl)
          n304 = Or(x=w1068, y=w1067) -> (x .or. y?=w1066:bool)
          n305 = Subtract(x=w1075, y=w1079) -> (x-y=w1074:dbl)
          n306 = for {
            tunnel: w1077 -> [w1091] mode=indexing
            tunnel: w1074 -> [w1092]
            tunnel: [w1090] -> w1076 mode=indexing
            tunnel: [w1089] -> w1073 mode=indexing
            n307 = Quotient & Remainder(x=w1092, y=w1091) -> (x-y*floor(x/y)=w1090:dbl, floor(x/y)=w1089:dbl)
          }
          n308 = Build Array (concatenate)(w1075, w1074, w1076) -> (w1063:dbl[])
          n309 = global write "GVZeitenZyklen.vi" "Big Ben, Methodenzeit, Zykluszeit0, Zykluszeit1, Zykluszeit2A, Zykluszeit2B"(w1063) -> ()
          n310 = To Long Integer(number=w1073) -> (32bit integer=w1062:i32[])
          n311 = global write "GVZeitenZyklen.vi" "ZyklusNummern"(w1062) -> ()
          n312 = Add(x=w1062, y=w1064) -> (x+y=w1061:i32[])
          n313 = Index Array(array=w1062, index=1 ("Index")) -> (element=w1071:i32)
          n314 = Add(x=w1071, y=w1070) -> (x+y=w1069:i32)
          n315 = global write "GVZeitenZyklen.vi" "ZyklusNummernGesamt"(w1061) -> ()
          n316 = call "Bis zum nächsten Vielfachen warten15"("Count(mSec)"=u32 50) -> ()  [unwired: 1 out]
        }
        n317 = Index Array(array=w744, index=3 ("Index")) -> (element=w742:dbl)
        n318 = while {
          tunnel: w792 -> [w819]
          tunnel: w791 -> [w818]
          tunnel: w707 -> [w833]
          shift-right: [w834] -> w783
          shift-left: w790 -> [w835]
          tunnel: w704 -> [w829]
          tunnel: w703 -> [w823]
          shift-right: [w820] -> _
          shift-left: w742 -> [w824]
          stop <- w836 stop-if-true
          n319 = global read "gvbooleschRT.vi" "global stop RT"() -> (w839:bool)
          n320 = local read "veränderte Methode benutzen"() -> (w837:bool)
          n321 = global read "GVMethodenwechsel.vi" "Methodenwechsel?"() -> (w838:bool)
          n322 = Compound Arithmetic op=OR(w839, w838, w837) -> (w836:bool)
          n323 = global read "GVZeitenZyklen.vi" "Big Ben, Methodenzeit, Zykluszeit0, Zykluszeit1, Zykluszeit2A, Zykluszeit2B"() -> (w831:dbl[])
          n324 = Index Array(array=w831, index=3 ("Index")) -> (element=w820:dbl)
          n325 = Greater Or Equal?(x=w820, y=w829) -> (x >= y?=w828:bool)
          n326 = Less?(x=w824, y=w829) -> (x < y?=w827:bool)
          n327 = Greater Or Equal?(x=w820, y=w823) -> (x >= y?=w826:bool)
          n328 = Less?(x=w824, y=w823) -> (x < y?=w825:bool)
          n329 = And(x=w826, y=w825) -> (x .and. y?=w822:bool)
          n330 = And(x=w828, y=w827) -> (x .and. y?=w817:bool)
          n331 = Or(x=w817, y=w822) -> (x .or. y?=w821:bool)
          n332 = And(x=w833, y=w821) -> (x .and. y?=w832:bool)
          n333 = case shown="True" w832 {
            tunnel: w835 -> [w841 w842]
            tunnel: [w841 w846] -> w834
            tunnel: w819 -> [_ w845]
            tunnel: w818 -> [_ w844]
            tunnel: w817 -> [_ w843]
            frame False {
            }
            frame True {
              n334 = call "MSDateienSchicken02-15.vi"("MSNummer"=w842, "MSa?"=w843, "Dateipfad:fromcriordy"=w844, "Dateipfad:fromcriocmd"=w845) -> ()  [unwired: 1 in]
              n335 = Increment(x=w842) -> (x+1=w846:i32)
            }
          }
          n336 = call "Bis zum nächsten Vielfachen warten13"("Count(mSec)"=u32 100 ("Zu wartende ms")) -> ()  [unwired: 1 out]
        }
        n337 = global read "gvbooleschRT.vi" "global stop RT"() -> (w798:bool)
      }
      n338 = case shown="True" "ECDSpeichern" {
        frame False {
        }
        frame True {
          w622 = dbl[] []
          n339 = global read "GVaktuelleTDMS.vi" "aktuelleTDMS-DateiECD1"() -> (w623:refnum<k34>)
          n340 = while {
            shift-right: [w631] -> _
            shift-left: w622 -> [w635]
            shift-right: [w624] -> _
            shift-left: w622 -> [w628]
            shift-right: [w630] -> _
            shift-left: w623 -> [w633]
            tunnel: w622 -> [w627]
            stop <- w640 stop-if-true
            n341 = call "Bis zum nächsten Vielfachen warten3"("Count(mSec)"=u32 500) -> ()  [unwired: 1 out]
            n342 = global read "GVaktuelleTDMS.vi" "aktuelleTDMS-DateiECD1"() -> (w630:refnum<k34>)
            n343 = global read "GVaktuelleTDMS.vi" "aktuelleTDMS-DateiECD2"() -> (w638:refnum<k34>)
            n344 = global read "GVECDs.vi" "ECD2MW"() -> (w625:dbl[])
            n345 = Build Array (concatenate)(w628, w625) -> (w629:dbl[])
            n346 = global read "GVECDs.vi" "ECD1MW"() -> (w634:dbl[])
            n347 = Build Array (concatenate)(w635, w634) -> (w632:dbl[])
            n348 = global read "gvbooleschRT.vi" "global stop RT"() -> (w640:bool)
            n349 = Equal?(x=w633, y=w630) -> (x = y?=w626:bool)
            n350 = TDMS Write(0:w630, 7:"ECD1", 9:w634) -> ()  [unwired: 3 in, 4 out]
            n351 = TDMS Write(0:w638, 7:"ECD2", 9:w625) -> ()  [unwired: 3 in, 4 out]
            n352 = Select(t=w632, s=w626, f=w627) -> (s? t:f=w631:dbl[])
            n353 = global write "GVChroms.vi" "ECD1Chrom"(w631) -> ()
            n354 = Select(t=w629, s=w626, f=w627) -> (s? t:f=w624:dbl[])
            n355 = global write "GVChroms.vi" "ECD2Chrom"(w624) -> ()
          }
        }
      }
      n356 = case shown="True" "HKSpeichern" {
        tunnel: w328 -> [_ w663]
        frame False {
        }
        frame True {
          n357 = while {
            tunnel: w663 -> [w677]
            stop <- w680 stop-if-true
            n358 = global read "GVZeitenZyklen.vi" "Big Ben, Methodenzeit, Zykluszeit0, Zykluszeit1, Zykluszeit2A, Zykluszeit2B"() -> (w668:dbl[])
            n359 = call "Bis zum nächsten Vielfachen warten2"("Count(mSec)"=u32 1000) -> ()  [unwired: 1 out]
            n360 = global read "GVZeitenZyklen.vi" "ZyklusNummernGesamt"() -> (w666:i32[])
            n361 = global read "GVHK1Hz.vi" "Mod1Mod2Mod3/AITrapsMachs1Hz"() -> (w672:dbl[])
            n362 = global read "GVZeitenZyklen.vi" "ZyklusNummern"() -> (w667:i32[])
            n363 = global read "GVProbenvol.vi" "Probenvol.1"() -> (w665:dbl)
            n364 = global read "GVProbenvol.vi" "Probenvol.2"() -> (w664:dbl)
            n365 = global read "GVaktuelleTDMS.vi" "aktuelleTDMS-DateiHK"() -> (w671:refnum<k34>)
            n366 = global read "GVMWHorst.vi" "MWHorst"() -> (w673:dbl[])
            n367 = Index Array(array=w666, index=1 ("Index")) -> (element=w669:i32)
            n368 = To Double Precision Float(number=w669) -> (double precision float=w675:dbl)
            n369 = To Double Precision Float(number=w667) -> (double precision float=w674:dbl[])
            n370 = global read "gvbooleschRT.vi" "global stop RT"() -> (w680:bool)
            n371 = Build Array (concatenate)(w675, w674, w668, w672, w673, w665, w664) -> (w676:dbl[])
            n372 = TDMS Write(0:w671, 1:enum16{"decimated", "interleaved"}."interleaved" ("Daten-Layout (0:dezimiert)"), 7:w677, 9:w676) -> ()  [unwired: 2 in, 4 out]
          }
        }
      }
      n373 = while {
        shift-right: [w333] -> _
        shift-left: w226 -> [w335]
        shift-right: [w332] -> _
        shift-left: w226 -> [w334]
        stop <- w337 stop-if-true
        n374 = call "Bis zum nächsten Vielfachen warten"("Count(mSec)"=u32 100) -> ()  [unwired: 1 out]
        n375 = global read "gvbooleschRT.vi" "global stop RT"() -> (w337:bool)
        n376 = case shown="True" "An/Aus" {
          tunnel: w335 -> [w339 w355]
          tunnel: w334 -> [w338 w354]
          tunnel: [w339 w348] -> w333
          tunnel: [w338 w347] -> w332
          frame False {
          }
          frame True {
            w351 = dbl[] [] ("t")
            n377 = global read "GVZeitenZyklen.vi" "Big Ben, Methodenzeit, Zykluszeit0, Zykluszeit1, Zykluszeit2A, Zykluszeit2B"() -> (w342:dbl[])
            n378 = global read "GVTrapsMachs.vi" "Traps/Machs"() -> (w345:dbl[])
            n379 = global read "GVMWHorst.vi" "MWHorst"() -> (w344:dbl[])
            n380 = Build Array (concatenate)(w345, w344) -> (w343:dbl[])
            n381 = Index Array(array=w343, index="dargestellte Größe 3") -> (element=w356:dbl)
            n382 = Build Array (concatenate)(w355, w356) -> (w349:dbl[])
            n383 = Index Array(array=w342, index=1 ("Index")) -> (element=w340:dbl)
            n384 = Build Array (concatenate)(w354, w340) -> (w350:dbl[])
            n385 = Bundle(w350, w349) -> (→"schnelleAnzeige":cluster{dbl[], dbl[]})  [unwired: 1 in]
            n386 = Select(t=w351, s="TafelWischen!", f=w349) -> (s? t:f=w348:dbl[])
            n387 = Select(t=w351, s="TafelWischen!", f=w350) -> (s? t:f=w347:dbl[])
          }
        }
      }
      n388 = Index Array(array=w249, index #1=0 ("Index"), index #2=1 ("Index"), index #3=2 ("Index"), index #4=3 ("Index")) -> (element #1=w290:i32, element #2=w289:i32, element #3=w292:i32, element #4=w291:i32)
      n389 = Add(x=w292, y=w291) -> (x+y=w288:i32)
      n390 = Build Array(w290, w289, w288) -> (w287:i32[])
      n391 = for {
        N: 1 -> [_]
        tunnel: w254 -> [w692]
        tunnel: [w692] -> w281
        n392 = call "Warten8"("Count(mSec)"=u32 100) -> ()  [unwired: 1 out]
      }
      n393 = Index Array(array=w287, index #1=0 ("Index"), index #2=1 ("Index")) -> (element #1=w308:i32, element #2=w306:i32)
      n394 = Split 1D Array(array=w284, index=w308) -> (first subarray=w315:string[], second subarray=w317:string[])
      n395 = Split 1D Array(array=w286, index=w308) -> (first subarray=w312:dbl[], second subarray=w316:dbl[])
      n396 = Split 1D Array(array=w285, index=w308) -> (first subarray=w305:string[], second subarray=w307:string[])
      n397 = call <vilib>:"Space Constant.vi"() -> ("String"=w232:string)
      n398 = Concatenate Strings("?SE0,GDATA" ("Schreibpuffer"), "\r") -> (w227:string)
      n399 = Add Array Elements(numeric array=w287) -> (sum=w297:i32)
      n400 = Split 1D Array(array=w316, index=w306) -> (first subarray=w311:dbl[], second subarray=w310:dbl[])
      n401 = Build Array(w232) -> (w231:string[])
      n402 = Split 1D Array(array=w317, index=w306) -> (first subarray=w314:string[], second subarray=w313:string[])
      n403 = Split 1D Array(array=w307, index=w306) -> (first subarray=w304:string[], second subarray=w303:string[])
      n404 = Initialize Array("x", 8 ("Dimension")) -> (w233:string[])
      n405 = global read "GVVentilposition.vi" "Ventilposition"() -> (w260:i32)
      n406 = Bundle(w315, w314, w313, w312, w311, w310) -> (w309:T21)  [unwired: 1 in]
      n407 = Initialize Array(0.0, 8 ("Dimension")) -> (w228:dbl[])
      n408 = Bundle(w305, w304, w303) -> (w302:cluster{string[], string[], string[]})  [unwired: 1 in]
      n409 = Bundle(w231, w231, w231) -> (w299:cluster{string[], string[], string[]})  [unwired: 1 in]
      n410 = Initialize Array(-1.0 ("Element"), w297) -> (w282:dbl[])
      n411 = Bundle(w301, w301, w301) -> (w300:cluster{i32, i32, i32})  [unwired: 1 in]
      n412 = case shown="True" "SerielleKomm." {
        tunnel: bool[] [TRUE, TRUE, TRUE, TRUE, TRUE, TRUE, TRUE, TRUE] -> [_ w397]
        tunnel: w233 -> [_ w396]
        tunnel: w309 -> [_ w395]
        tunnel: w308 -> [_ w394]
        tunnel: w306 -> [_ w393]
        tunnel: w302 -> [_ w392]
        tunnel: w300 -> [_ w391]
        tunnel: w299 -> [_ w390]
        tunnel: w286 -> [_ w389]
        tunnel: w283 -> [_ w388]
        tunnel: w282 -> [_ w387]
        tunnel: w281 -> [_ w384]
        tunnel: w260 -> [_ w386]
        tunnel: w228 -> [_ w385]
        tunnel: w227 -> [_ w383]
        frame False {
        }
        frame True {
          n413 = while {
            shift-right: [w567] -> _
            shift-left: w397 -> [w542]
            shift-right: [w550] -> _
            shift-left: w387 -> [w562]
            tunnel: w384 -> [w549]
            shift-right: [w540] -> _
            shift-left: w396 -> [w566]
            tunnel: w388 -> [w565]
            tunnel: w389 -> [w564]
            shift-right: [w552] -> _
            shift-left: w390 -> [w554]
            tunnel: w394 -> [w560]
            tunnel: w393 -> [w561]
            tunnel: w395 -> [w563]
            tunnel: w392 -> [w557]
            shift-right: [w556] -> _
            shift-left: w391 -> [w558]
            shift-right: [w546] -> _
            shift-left: w386 -> [w548]
            shift-right: [w543] -> _
            shift-left: w385 -> [w544]
            stop <- w551 stop-if-true
            n414 = for {
              tunnel: w542 -> [w571] mode=indexing
              tunnel: w544 -> [w568] mode=indexing
              tunnel: [w575] -> w543 mode=indexing
              tunnel: [w572] -> w541 mode=indexing
              n415 = global read "GVZeitenZyklen.vi" "Big Ben, Methodenzeit, Zykluszeit0, Zykluszeit1, Zykluszeit2A, Zykluszeit2B"() -> (w578:dbl[])
              n416 = Index Array(array=w578, index=0 ("Index")) -> (element=w576:dbl)
              n417 = Subtract(x=w576, y=w568) -> (x-y=w574:dbl)
              n418 = Greater?(x=w574, y=0.1) -> (0:w570:bool)
              n419 = Or(x=w571, y=w570) -> (x .or. y?=w569:bool)
              n420 = Select(t=w570, s=w570, f=w571) -> (s? t:f=w572:bool)
              n421 = Select(t=w576, s=w569, f=w568) -> (s? t:f=w575:dbl)
            }
            n422 = global read "GVHorstSP.vi" "HorstSP"() -> (w550:dbl[])
            n423 = call "Warten3"("Count(mSec)"=u32 10) -> ()  [unwired: 1 out]
            n424 = Not Equal?(x=w550, y=w562) -> (x != y?=w555:bool)
            n425 = call "NeueSP.vi"("Anzahl2"=w561, "Anzahl1"=w560, "AlteSP"=w562, 7:"NeueSP"=w550, "BefehleCluster"=w554, 10:"NeueSP"=w555, "ClusterFest"=w563) -> ("BefehleCluster"=w553:T22)  [unwired: 4 in]
            n426 = call "MPVSenden.vi"("Ventilposition"=w548, "FPGA VI Reference"=w549) -> ("Ventilposition"=w546:i32, "FPGA VI Reference"=w547:refnum<k20>)
            n427 = call "Senden.vi"("FPGA VI Reference In"=w547, "BefehlsCluster"=w553, "Senden?"=w541, "Abfragenr.Cluster"=w558, "AbfragenCluster"=w557) -> ("Senden?"=w559:bool[], "Abfragenr.Cluster"=w556:cluster{i32, i32, i32}, "BefehlsCluster"=w552:T22)  [unwired: 1 in]
            n428 = call "SeriellRead.vi"("SkalierungsfaktorHorst"=w564, "VorwortHorst"=w565, "Zwischenspeicher"=w566, "Senden?"=w559, "FPGA VI Reference In"=w547) -> ("Senden?"=w567:bool[], "Zwischenspeicher"=w540:string[])  [unwired: 5 in]
            n429 = global read "gvbooleschRT.vi" "global stop RT"() -> (w551:bool)
          }
          n430 = while {
            tunnel: w384 -> [w405]
            tunnel: w383 -> [w404]
            stop <- w407 stop-if-true
            n431 = String To Byte Array(string=w404) -> (unsigned byte array=w400:u8[])
            n432 = Join Numbers(hi=w400, lo=u8 5) -> ((hi.lo)=w402:u16[])
            n433 = call "Warten6"("Count(mSec)"=u32 500) -> ()  [unwired: 1 out]
            n434 = xnode "Invoke Method"("FPGA VI Reference In"=w405, "Data"=w402) -> ("FPGA VI Reference Out"=w401:refnum<k20>)  [unwired: 2 in, 2 out]
            n435 = Join Numbers(hi=w400, lo=u8 6) -> ((hi.lo)=w398:u16[])
            n436 = xnode "Invoke Method"("FPGA VI Reference In"=w401, "Data"=w398) -> ()  [unwired: 2 in, 3 out]
            n437 = global read "gvbooleschRT.vi" "global stop RT"() -> (w407:bool)
          }
        }
      }
      n438 = Unbundle(w275) -> ("Dateiordner Housekeeping"=w274:path, "DateiordnerECD1"=w272:path, "DateiordnerECD2"=w271:path, "Dateiname Housekeeping"=w273:string, "DateinameECD1"=w270:string, "DateinameECD2"=w269:string, "tdms0"=w268:refnum<k34>, "tdms1"=w267:refnum<k34>, "tdms0"=w266:refnum<k34>, "tdms1"=w265:refnum<k34>, "tdms0"=w264:refnum<k34>, "tdms1"=w263:refnum<k34>)
      n439 = local read "HKSpeichern"() -> (w239:bool)
      n440 = case shown="True" w239 {
        tunnel: w276 -> [_ w647]
        tunnel: w274 -> [_ w646]
        tunnel: w273 -> [_ w645]
        tunnel: w268 -> [_ w644]
        tunnel: w267 -> [_ w643]
        frame False {
        }
        frame True {
          n441 = while {
            shift-right: [w655] -> w642
            shift-left: w644 -> [w649]
            shift-right: [w659] -> w641
            shift-left: w643 -> [w651]
            shift-right: [w653] -> _
            shift-left: w647 -> [w660]
            tunnel: w645 -> [w656]
            tunnel: w646 -> [w657]
            stop <- w662 stop-if-true
            n442 = global read "GVZeitenZyklen.vi" "ZyklusNummernGesamt"() -> (w648:i32[])
            n443 = call "Bis zum nächsten Vielfachen warten5"("Count(mSec)"=u32 500) -> ()  [unwired: 1 out]
            n444 = Index Array(array=w648, index=1 ("Index")) -> (element=w653:i32)
            n445 = Greater?(x=w653, y=w660) -> (0:w652:bool)
            n446 = Select(t=w651, s=w652, f=w649) -> (s? t:f=w650:refnum<k34>)
            n447 = global write "GVaktuelleTDMS.vi" "aktuelleTDMS-DateiHK"(w650) -> ()
            n448 = local read "Methode"() -> (w658:i32)
            n449 = global read "gvbooleschRT.vi" "global stop RT"() -> (w662:bool)
            n450 = call "AktuelleTDMS.vi"("AktuelleTDMS"=w649, "Dateiordner"=w657, "NächsteTDMS"=w651, "NeuerZyklus?"=w652, "Methodennummer"=w658, "Zyklnumges"=w653, "Dateiname"=w656) -> ("AktuelleTDMS"=w655:refnum<k34>, "NächsteTDMS"=w659:refnum<k34>)  [unwired: 5 in, 2 out]
          }
          n451 = TDMS Close(11:w642) -> ()  [unwired: 1 in, 2 out]
          n452 = TDMS Close(11:w641) -> ()  [unwired: 1 in, 2 out]
        }
      }
      n453 = local read "ECDSpeichern"() -> (w237:bool)
      n454 = case shown="True" w237 {
        tunnel: w276 -> [_ w591]
        tunnel: w272 -> [_ w590]
        tunnel: w271 -> [_ w589]
        tunnel: w270 -> [_ w588]
        tunnel: w269 -> [_ w587]
        tunnel: w266 -> [_ w586]
        tunnel: w265 -> [_ w585]
        tunnel: w264 -> [_ w584]
        tunnel: w263 -> [_ w583]
        frame False {
        }
        frame True {
          n455 = while {
            shift-right: [w616] -> w582
            shift-left: w586 -> [w608]
            shift-right: [w617] -> w581
            shift-left: w585 -> [w610]
            shift-right: [w614] -> _
            shift-left: w591 -> [w618]
            tunnel: w590 -> [w613]
            tunnel: w588 -> [w612]
            stop <- w620 stop-if-true
            n456 = global read "GVZeitenZyklen.vi" "ZyklusNummernGesamt"() -> (w607:i32[])
            n457 = call "Bis zum nächsten Vielfachen warten4"("Count(mSec)"=u32 500) -> ()  [unwired: 1 out]
            n458 = Index Array(array=w607, index=2 ("Index")) -> (element=w614:i32)
            n459 = Greater?(x=w614, y=w618) -> (0:w611:bool)
            n460 = Select(t=w610, s=w611, f=w608) -> (s? t:f=w609:refnum<k34>)
            n461 = global write "GVaktuelleTDMS.vi" "aktuelleTDMS-DateiECD1"(w609) -> ()
            n462 = local read "Methode"() -> (w615:i32)
            n463 = global read "gvbooleschRT.vi" "global stop RT"() -> (w620:bool)
            n464 = call "AktuelleTDMS.vi"("AktuelleTDMS"=w608, "Dateiordner"=w613, "NächsteTDMS"=w610, "NeuerZyklus?"=w611, "Methodennummer"=w615, "Zyklnumges"=w614, "Dateiname"=w612) -> ("AktuelleTDMS"=w616:refnum<k34>, "NächsteTDMS"=w617:refnum<k34>)  [unwired: 5 in, 2 out]
          }
          n465 = while {
            shift-right: [w601] -> w580
            shift-left: w584 -> [w593]
            shift-right: [w602] -> w579
            shift-left: w583 -> [w595]
            shift-right: [w599] -> _
            shift-left: w591 -> [w603]
            tunnel: w589 -> [w598]
            tunnel: w587 -> [w597]
            stop <- w605 stop-if-true
            n466 = global read "GVZeitenZyklen.vi" "ZyklusNummernGesamt"() -> (w592:i32[])
            n467 = call "Bis zum nächsten Vielfachen warten6"("Count(mSec)"=u32 500) -> ()  [unwired: 1 out]
            n468 = Index Array(array=w592, index=3 ("Index")) -> (element=w599:i32)
            n469 = Greater?(x=w599, y=w603) -> (0:w596:bool)
            n470 = Select(t=w595, s=w596, f=w593) -> (s? t:f=w594:refnum<k34>)
            n471 = global write "GVaktuelleTDMS.vi" "aktuelleTDMS-DateiECD2"(w594) -> ()
            n472 = local read "Methode"() -> (w600:i32)
            n473 = global read "gvbooleschRT.vi" "global stop RT"() -> (w605:bool)
            n474 = call "AktuelleTDMS.vi"("AktuelleTDMS"=w593, "Dateiordner"=w598, "NächsteTDMS"=w595, "NeuerZyklus?"=w596, "Methodennummer"=w600, "Zyklnumges"=w599, "Dateiname"=w597) -> ("AktuelleTDMS"=w601:refnum<k34>, "NächsteTDMS"=w602:refnum<k34>)  [unwired: 5 in, 2 out]
          }
          n475 = TDMS Close(11:w581) -> ()  [unwired: 1 in, 2 out]
          n476 = TDMS Close(11:w582) -> ()  [unwired: 1 in, 2 out]
          n477 = TDMS Close(11:w580) -> ()  [unwired: 1 in, 2 out]
          n478 = TDMS Close(11:w579) -> ()  [unwired: 1 in, 2 out]
        }
      }
    }
    frame #2 {
      n479 = xnode "Read/Write Control"("FPGA VI Reference In"=w1195, "global stop"=TRUE) -> ("FPGA VI Reference Out"=w1194:refnum<k20>)  [unwired: 1 in, 1 out]
      n480 = xnode "Close FPGA VI Reference"("FPGA VI Reference In"=w1194) -> ()  [unwired: 1 in, 1 out]
    }
  }
  n481 = Open/Create/Replace File(file path (use dialog)=path "c:/methoden.per" ("Datei (Dialog verwenden)"), operation (0:open)=T4."open" ("Operation (0:Öffnen)")) -> (refnum out=w6:refnum<file>)  [unwired: 4 in, 2 out]
  n482 = Read from Binary File(5:T2 [] ("Methoden"), 11:w6) -> (2:w3:T2, 3:w5:refnum<file>)  [unwired: 4 in, 2 out]
  n483 = Close File(refnum=w5) -> ()  [unwired: 1 in, 2 out]
